vi "r3_Ladder bias ring encapsulation v1.vi"() -> ()   [LabVIEW 2016]
uses:
  WTF is this.ctl
  Classes/Controllers/I-O/Copy of NI-DAQ Folder/NI-DAQ.lvclass
  D:/INTT/V1/Classes/Controllers/I-O/Copy of I-O Folder/I-O.lvclass
  Classes/Controllers/Dispenser/Copy of Ultimus V2 Folder/Ultimus V2.lvclass
  <vilib>/Analysis/coordinate.llb/2D Cartesian Coordinate Rotation (Scalar).vi
  <vilib>/Utility/file.llb/Read Delimited Spreadsheet (DBL).vi
  <vilib>/Utility/file.llb/Write Delimited Spreadsheet (DBL).vi
  Classes/Controllers/Motion/Copy of Motion Folder/Motion.lvclass
  Classes/Controllers/Camera/Copy of Controller Folder/Controller.lvclass
  <vilib>/Analysis/NI_AALPro.lvlib
  Classes/Controllers/I-O/Copy of I-O Folder/I-O.lvclass
panel:
  in  "Needle gap for real":dbl=1.3
  out "corner index":i32
  out "Array":dbl[](array[numeric])
  out "x+y":dbl[](array[numeric])
  out "South":dbl[][][](array[numeric])
  out "North":dbl[][][](array[numeric])
  in  "deposit module":i32=2
  out "file indicator":dbl[][](array[numeric])
  out "?":dbl[](array[numeric]) format="%#_8g"
  in  "offset":dbl[](array[numeric])=[0.0, 0.0, 0.0, 0.0] format="%#_8g"
  out "HDI center positions":dbl[][](array[numeric]) format="%#_8g"
  out "HDI center positions":dbl[][](array[numeric])=[[459.92445114002015, 980.2358762511564, 78.77350133595746, 0.0015214873297426886]] format="%#_8g"
  out "CT sum up":dbl[](array[numeric])
  in  "txt switch":bool
  in  "MPT offset":dbl[][](array[numeric])=[[0.0, 0.0, 0.0, 0.0], [0.0, 0.0, 0.0, 0.0]] format="%#_8g"
  out "CT HPoS":dbl[][](array[numeric]) format="%#_8g"
  out "chip distance by OGP":dbl format="%#_8g"
  out "displacement":dbl[](array[numeric])
  out "gantry position test":dbl[](array[numeric])
  out "gantry target position":dbl[](array[numeric])
  out "chip distance by gantry":dbl format="%#_8g"
  out "after SL":dbl[](array[numeric]) format="%#_8g"
  out "after SR":dbl[](array[numeric]) format="%#_8g"
  out "after NL":dbl[](array[numeric]) format="%#_8g"
  out "S chip":dbl[](array[numeric]) format="%#_8g"
  out "N chip":dbl[](array[numeric]) format="%#_8g"
  in  "?":path=path "C:/Users/PAGANIS/Desktop/shih cheng wei/OGP/test1-2.txt"
  out "bless from OGP !!! Center of  stave":dbl[](array[numeric])
  out "bless from OGP !! measured stave size":dbl[](array[numeric])
  in  "Bless from OGP":bool
  out "FROM Detail !!! Center of module on stave":dbl[](array[numeric])
  out "FROM Detail !! measured stave size":dbl[](array[numeric])
  in  "Align Stave in detail":bool
  in  "check height?":bool
  in  "Uttimus presssure":i64=10
  out "Status":bool
  out "measured HDI top-left position":dbl[][](array[numeric])
  in  "HDI vacuum channel":i32=18
  in  "vacuum":bool=TRUE
  in  "HDI vacuum":bool
  out "measured stave size":dbl[](array[numeric])
  out "Stave mark":dbl[][](array[numeric])
  out "Center of module on stave":dbl[](array[numeric])
  out "Measured HDI size":dbl[][](array[numeric])
  out "MPT positions on stave":T1[][](array[typedef])
  in  "Default Stave dimension":dbl[](array[numeric])=[34.0, 472.0, -0.335295, -0.000320234]
  in  "Default Stave upper left mark":dbl[](array[numeric])=[584.376, 675.576, 70.9882, 0.000840064]
  out "Needle parking position":dbl[](array[numeric])
  in  "Uppler / Lower Stave":bool=TRUE
  out "Gantry current position":dbl[](array[numeric])
  in  "READ Position":bool
  in  "Needle Height Compenstation\n(glue gap)":dbl=0.33
  in  "Needle Alignment":bool
  in  "Parking position":dbl[](array[numeric])=[625.0, 625.0, 0.0, 0.01]
  in  "GOTO":bool
  in  "Default Pickup Tool Position":dbl[][](array[numeric])=[[152.226, 682.729, 36.8129, -0.0151898], [700.0, 800.0, 20.0, 0.01]]
  in  "deposit glue module":i32=1
  in  "Default HDI alignment \nmark position":dbl[](array[numeric])=[589.244, 676.291, 66.3411, 0.000190613]
  in  "Default HDI size":dbl[](array[numeric])=[24.2437, 231.446, -0.099339, 0.000191129]
  out "# of tasks excuted":i32
  out "PickupTool \nCenterPosition":dbl[](array[numeric]) format="%#_8g"
  in  "Inititalize":bool
  in  "Pick and place":bool
  in  "Deposit Glue":bool
  in  "Measure Pickup Tools":bool
  in  "Align Stave":bool
  out "default module position on stave":dbl[][](array[numeric])
  in  "Stop":bool
  in  "Measure HDI":bool
  # "Ladder Assembly"
  # "To switch the north/south\ntxt file \nswitch \noffset\nmodule pick up tool\nmodule direction"
  # "Upper\nmodule"
  # "Lower\nmodule"
  # "Sensor 0.32 -> 200 micron glue thickness\nChips 0.37-> 140 micron glue thickness"
  # "ACTIONS"
  # "theta had *-1"
  # "Pick up tool and needle"
  # "Module infomation"
  # "Pick and Place"
  # "CT"
  # "+"
  # "+"
  # "="
  # "Bias ring encapsulation"
  # "before \"HDI cornrer\" click \"Initialize\""
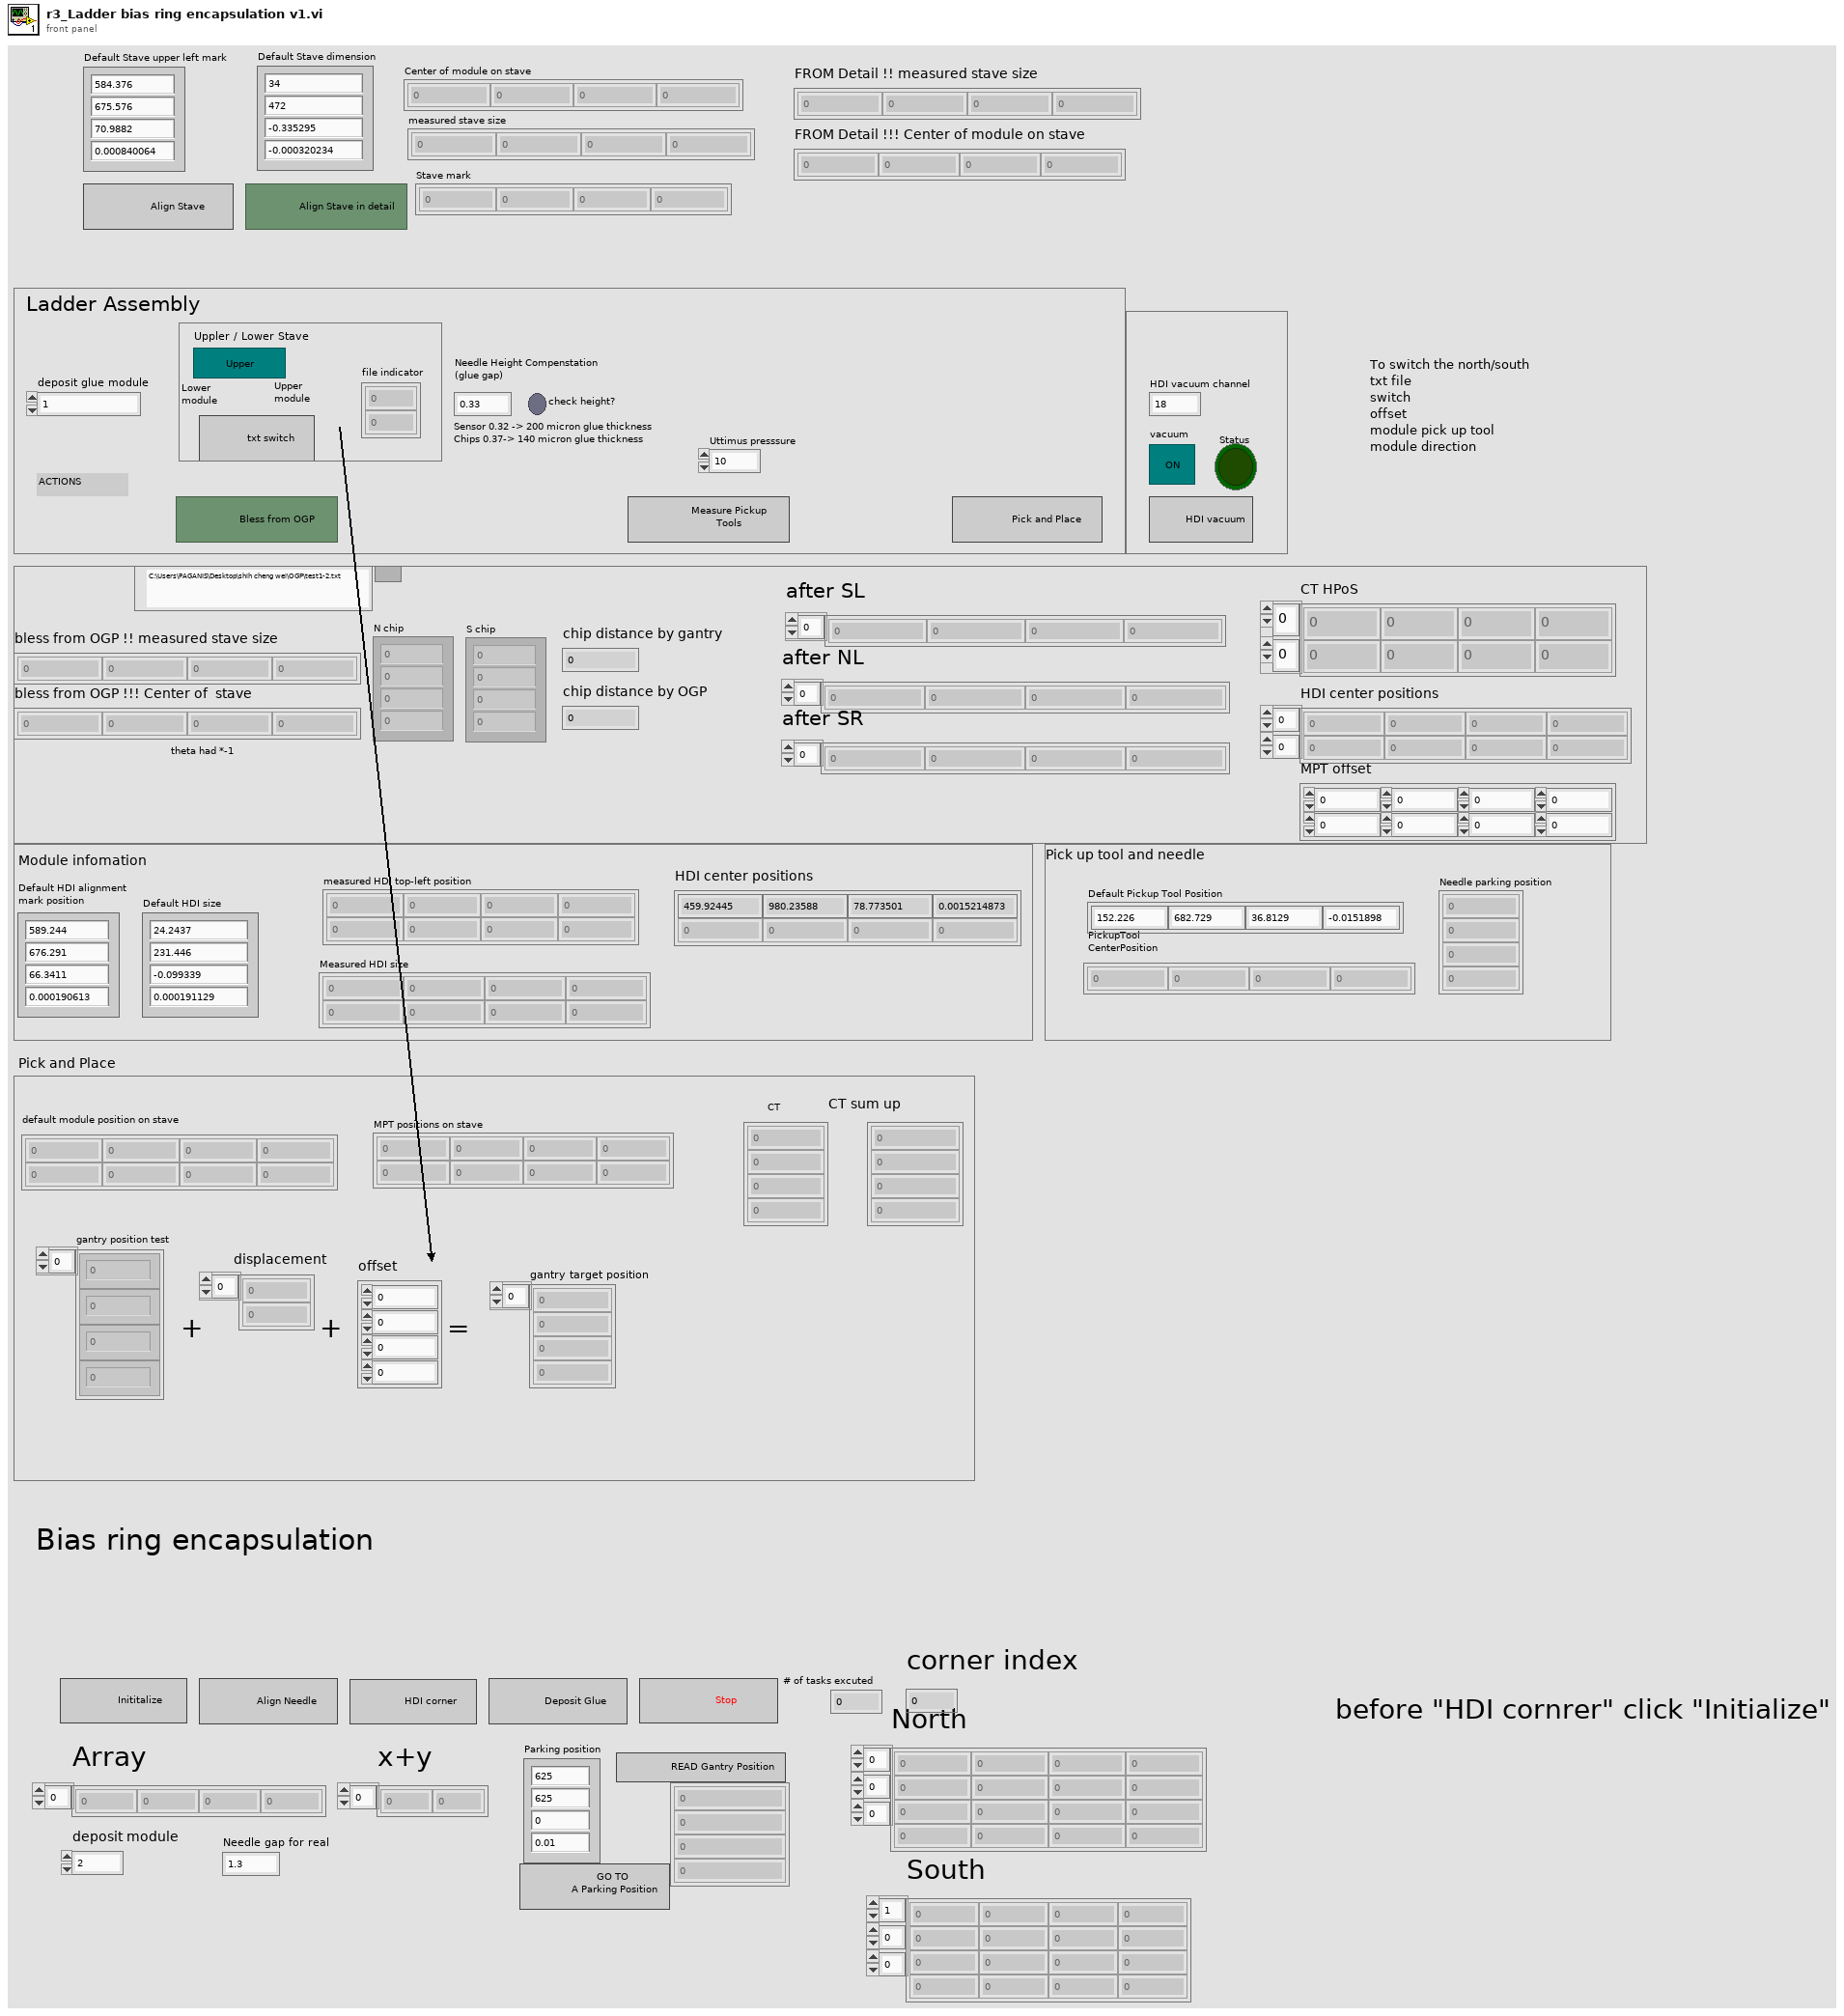
[diagram p1: front panel]
types:
  T1 = typedef "WTF is this.ctl" = dbl
  T2 = typedef "Controller.lvclass/Controllers.ctl" = cluster{"Copy of Motion.lvclass":refnum<class "Motion.lvclass">, "Copy of I-O.lvclass":refnum<class "I-O.lvclass">, "Copy of Dispenser.lvclass":refnum<class "Dispenser.lvclass">}
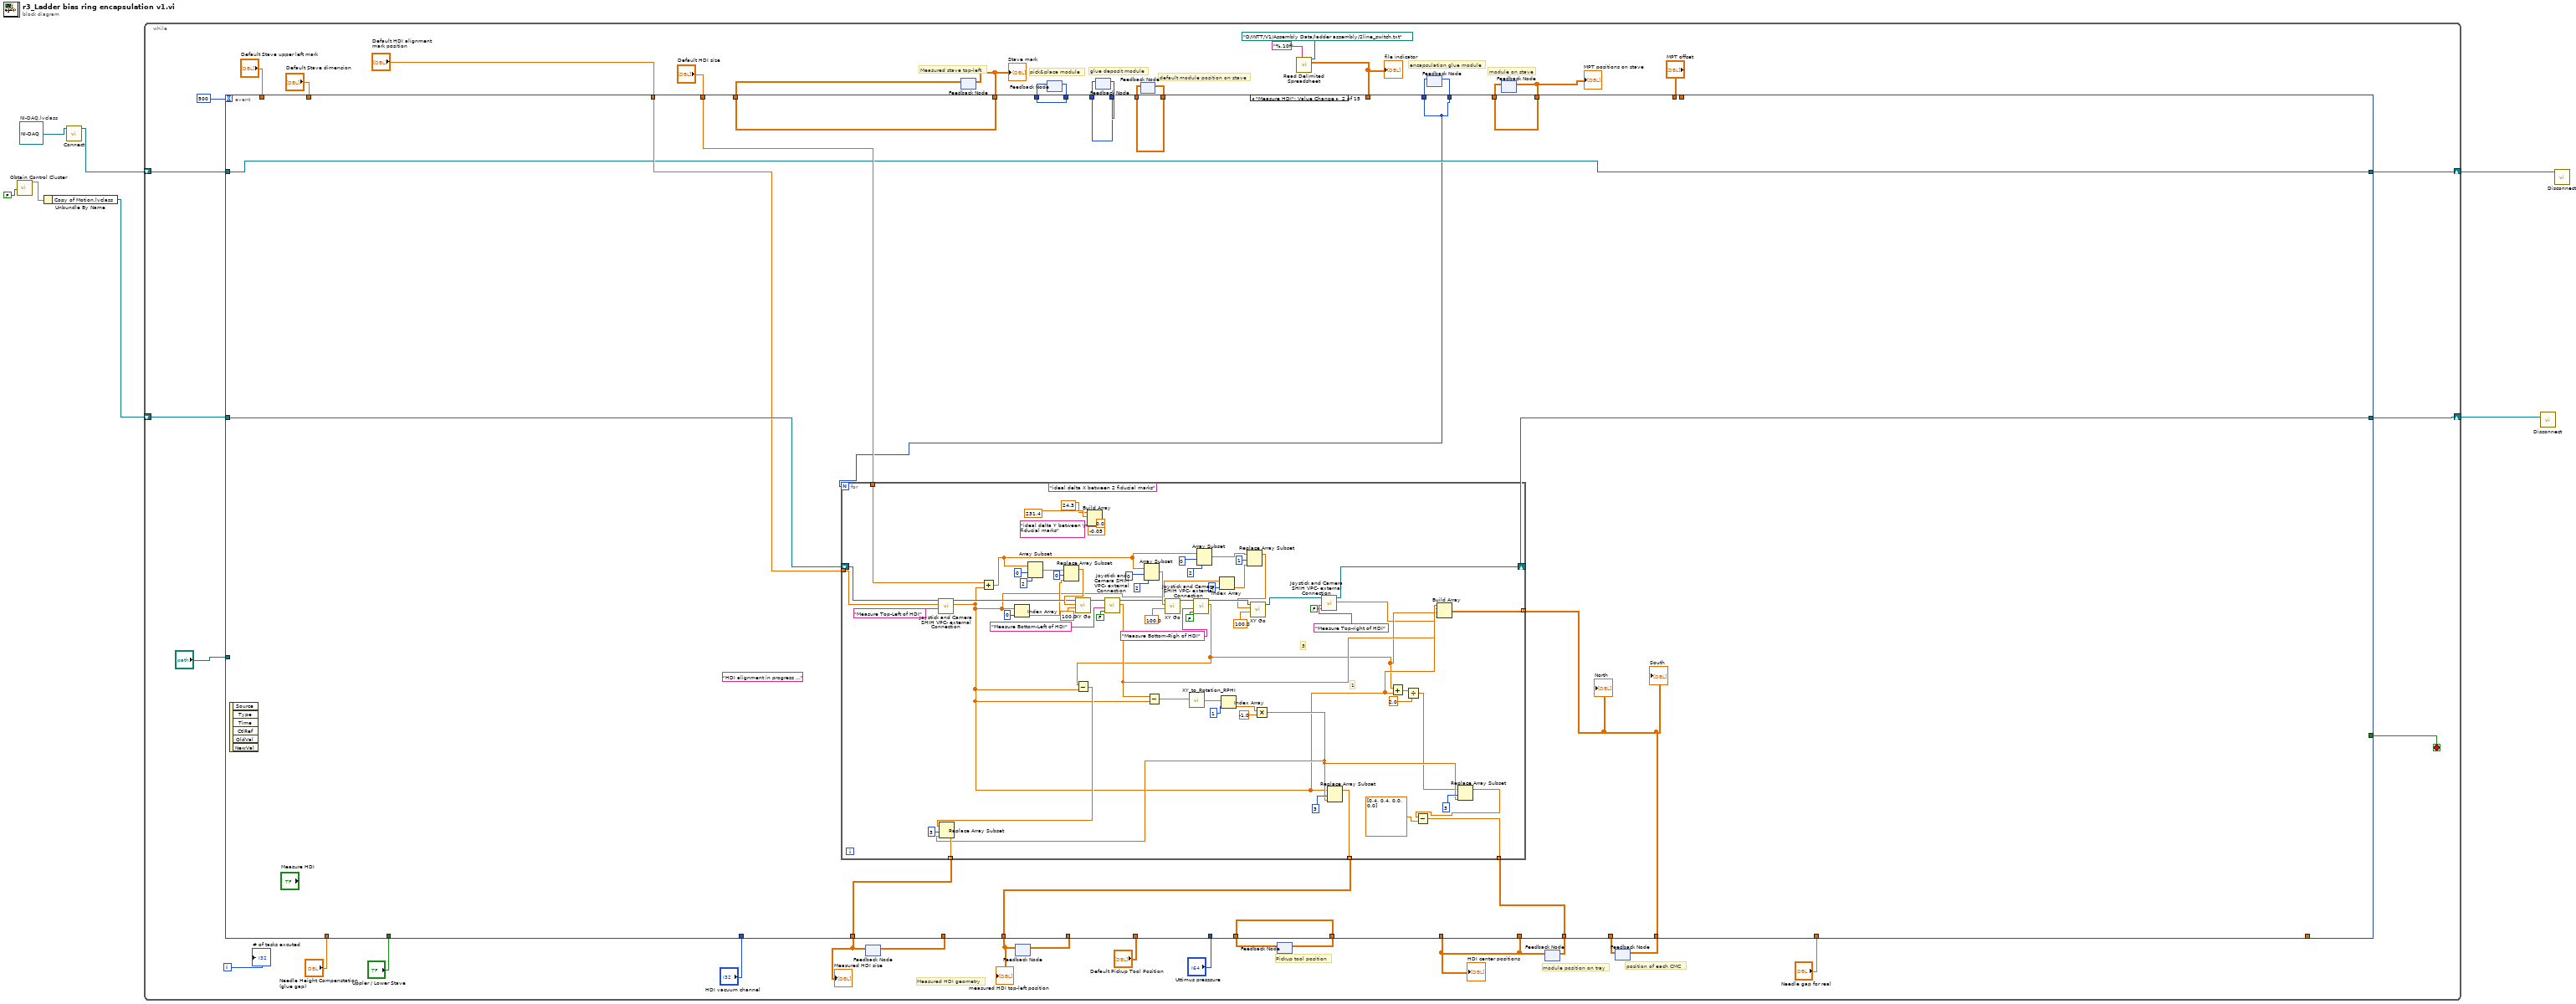
[diagram p0: block diagram]
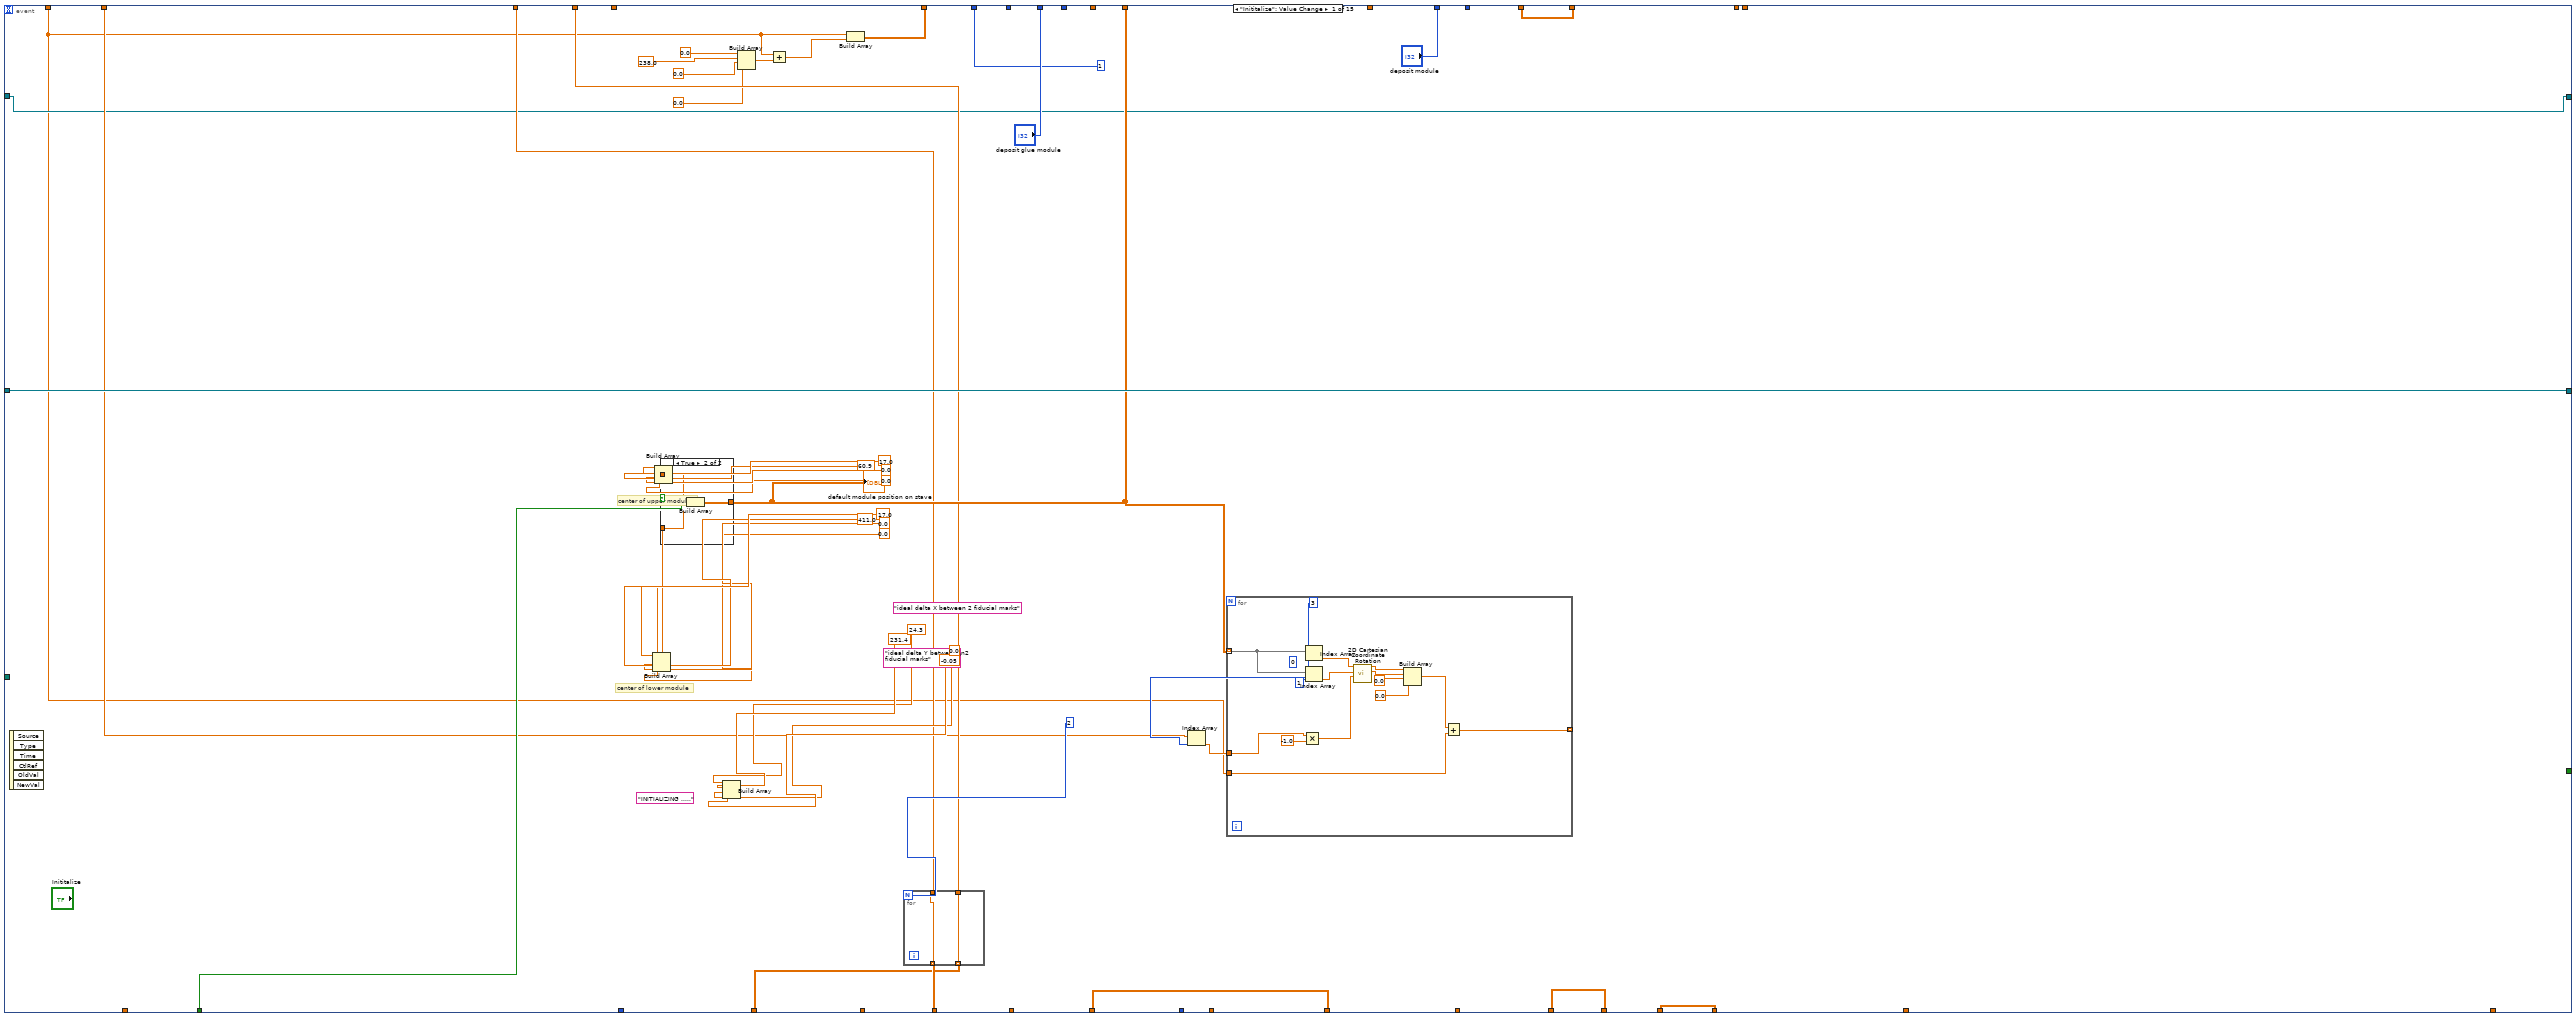
[diagram p2: hidden frame]
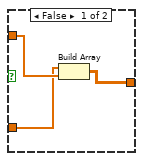
[diagram p3: hidden frame]
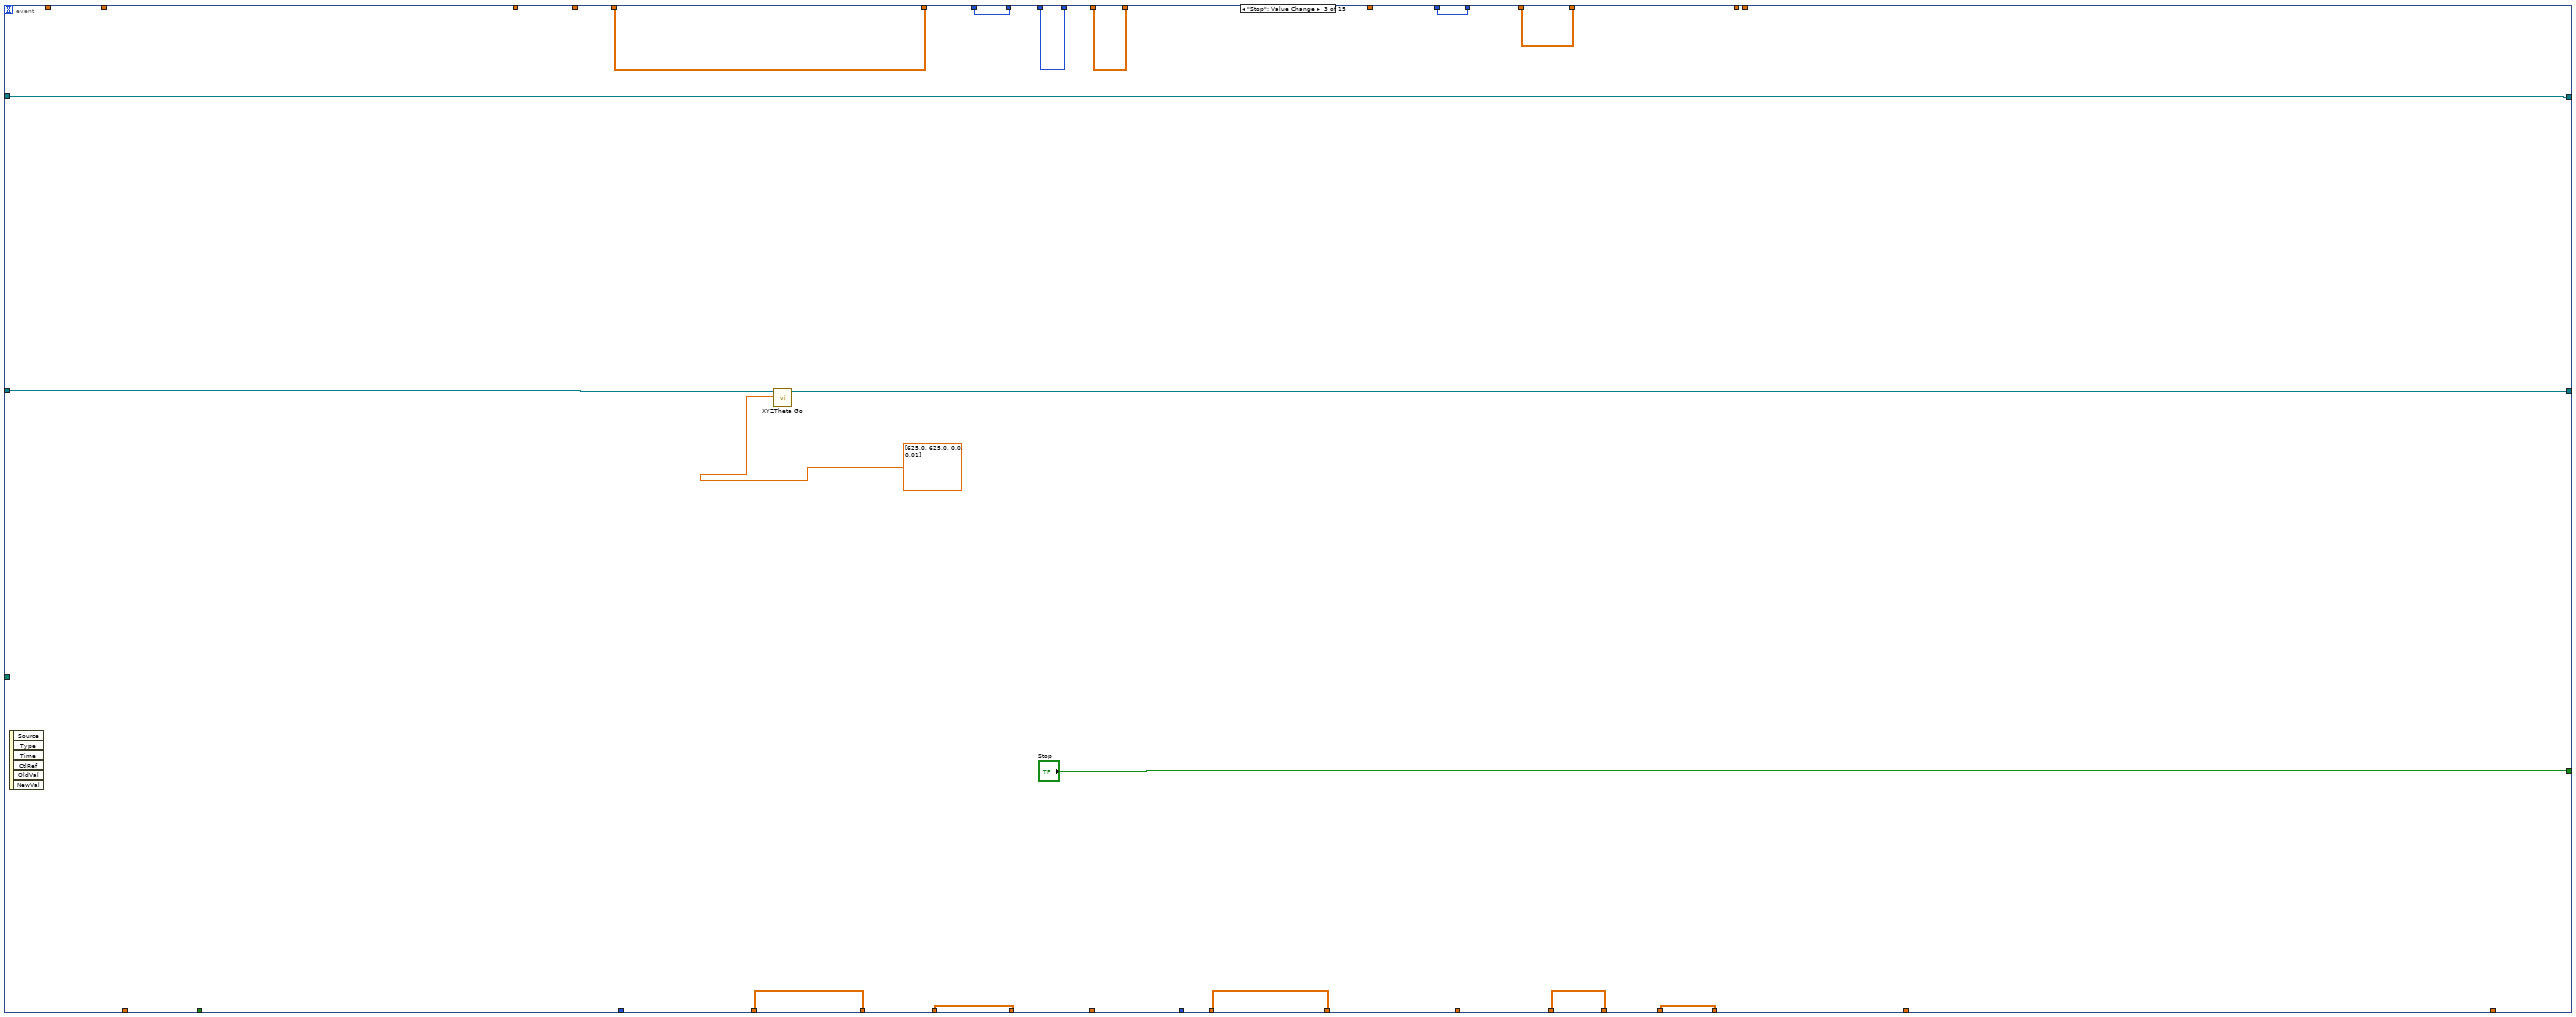
[diagram p4: hidden frame]
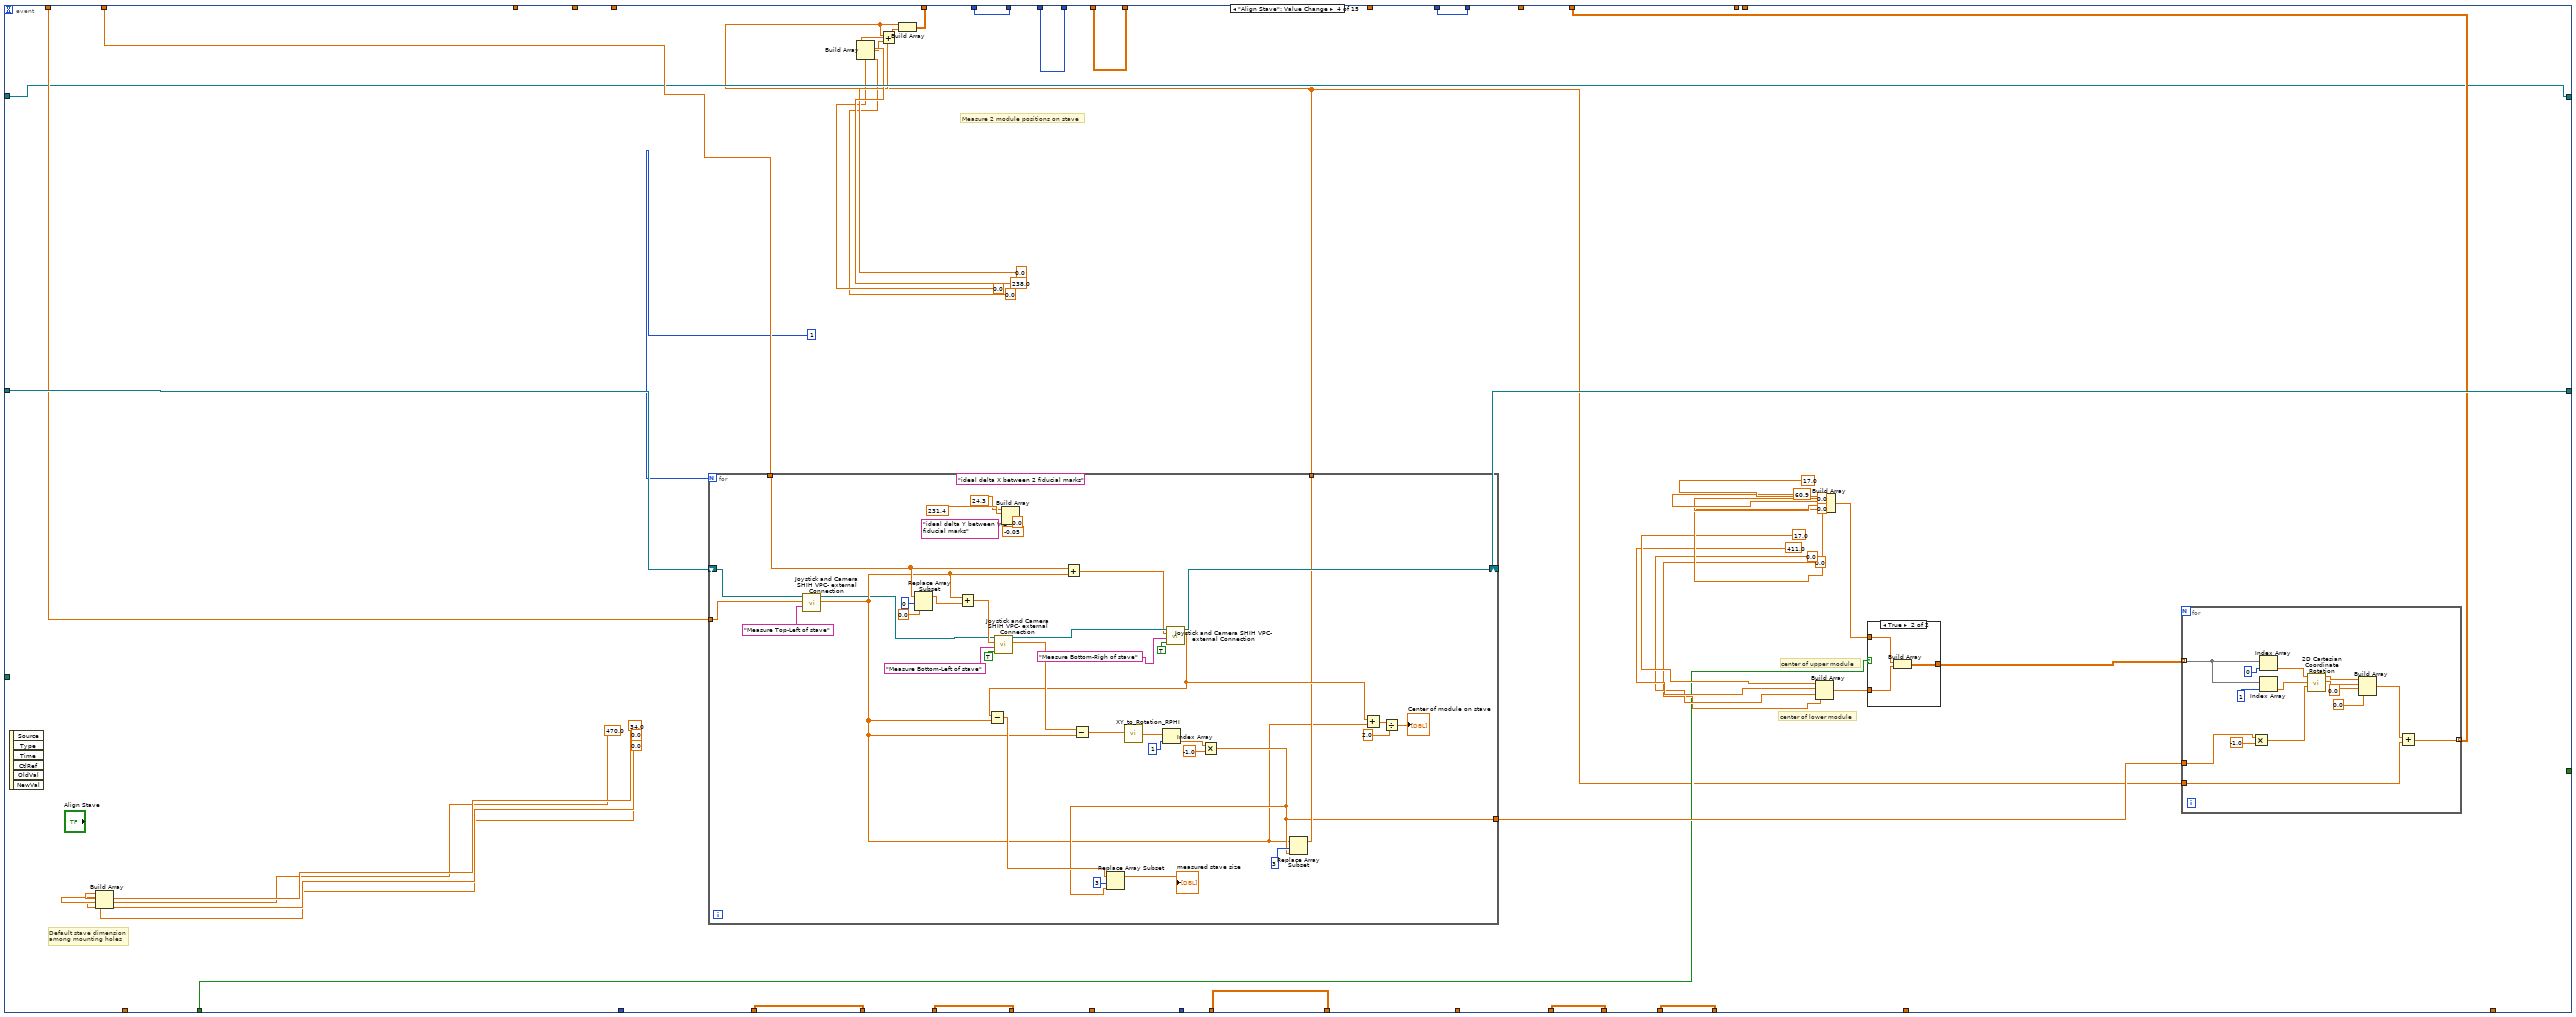
[diagram p5: hidden frame]
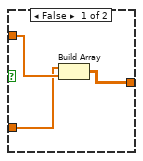
[diagram p6: hidden frame]
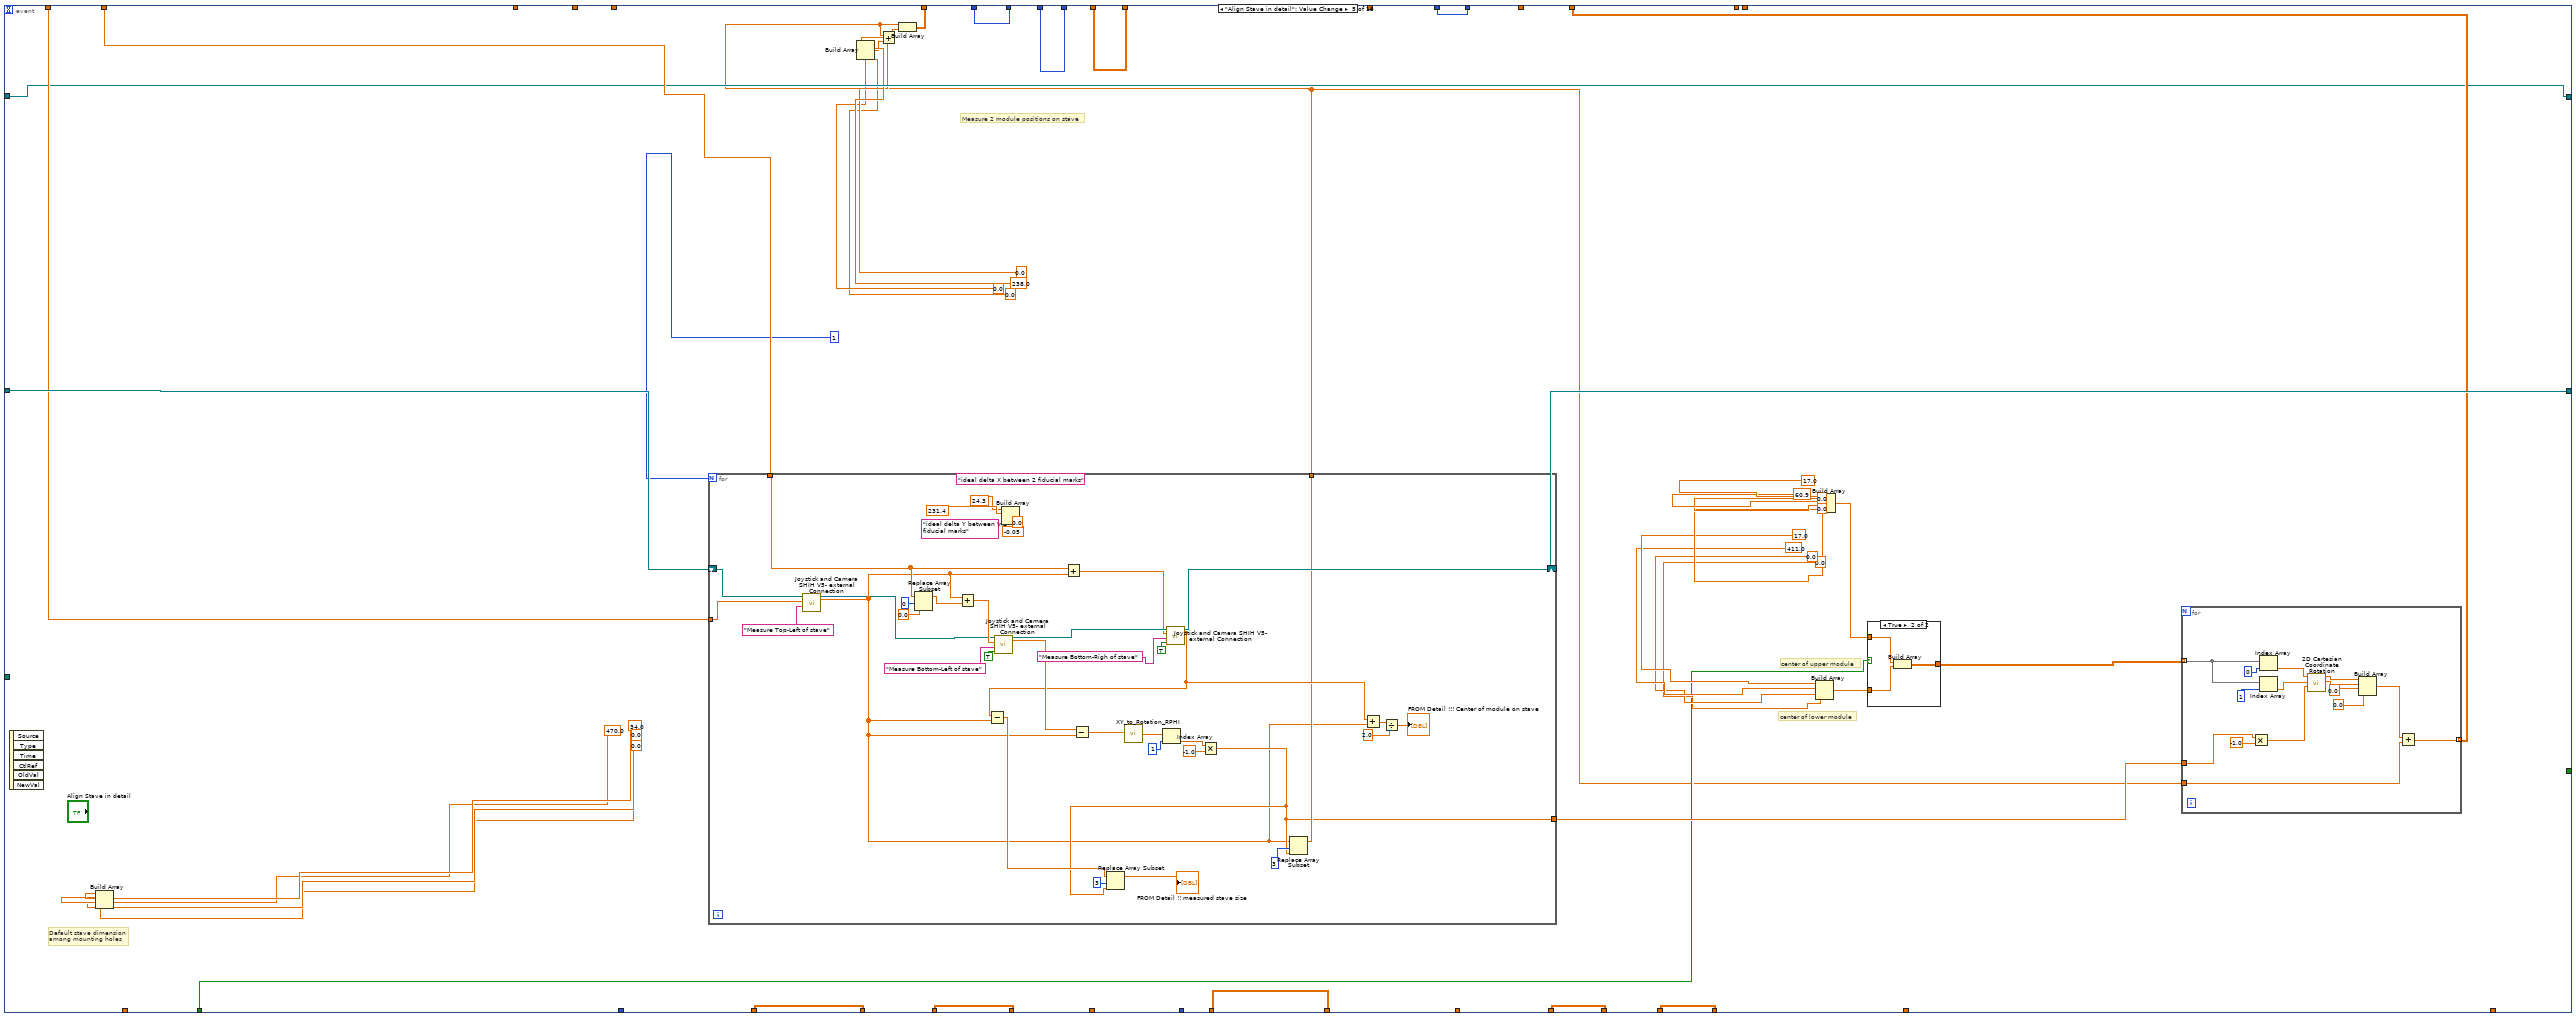
[diagram p7: hidden frame]
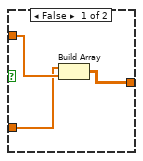
[diagram p8: hidden frame]
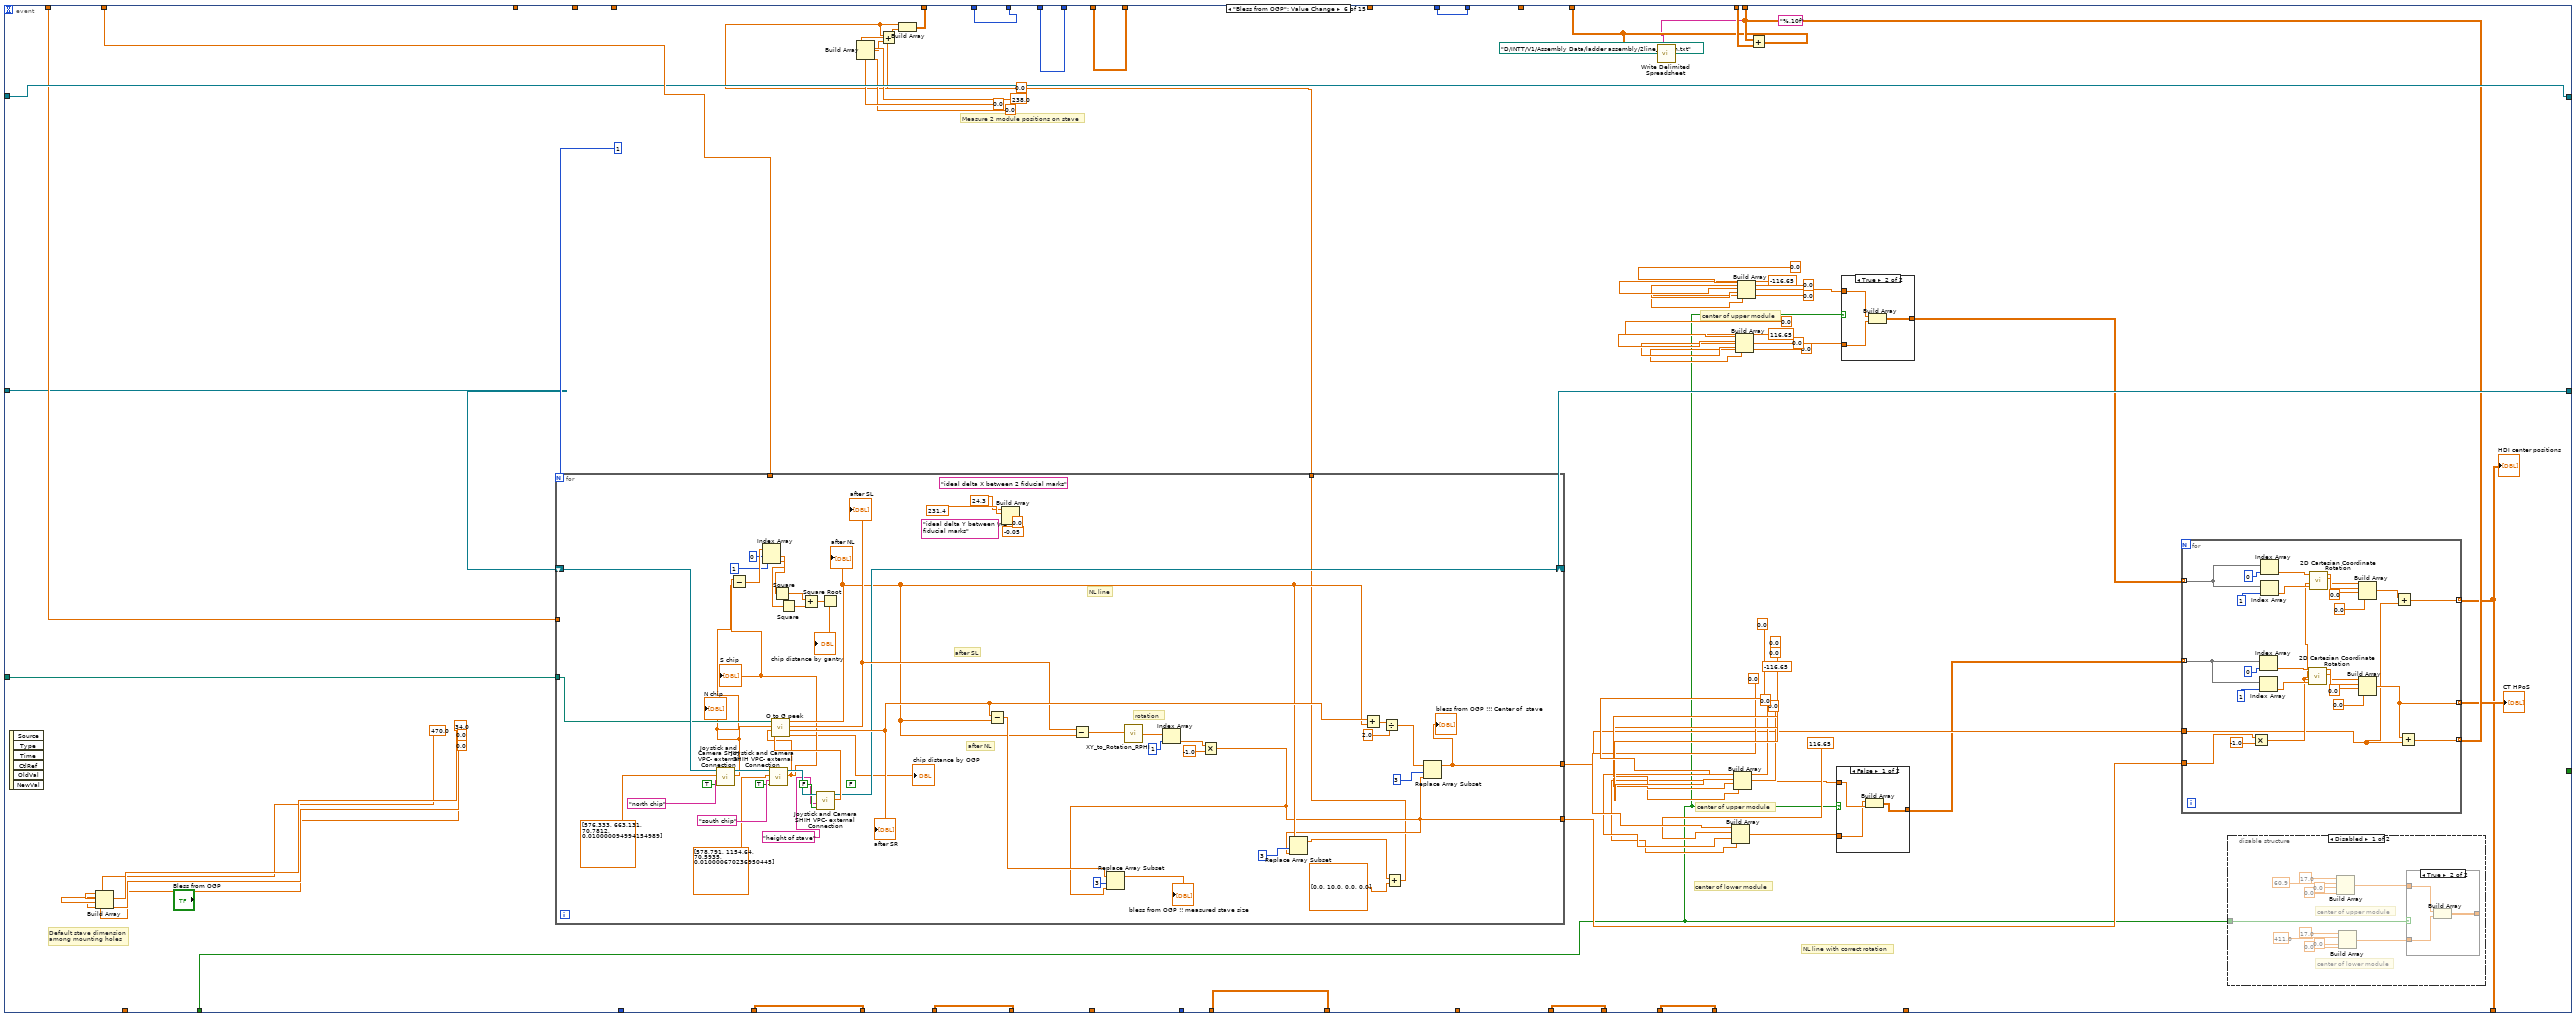
[diagram p9: hidden frame]
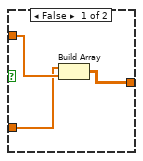
[diagram p10: hidden frame]
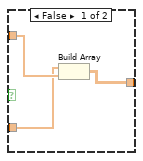
[diagram p11: hidden frame]
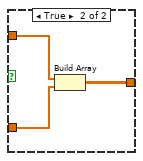
[diagram p13: hidden frame]
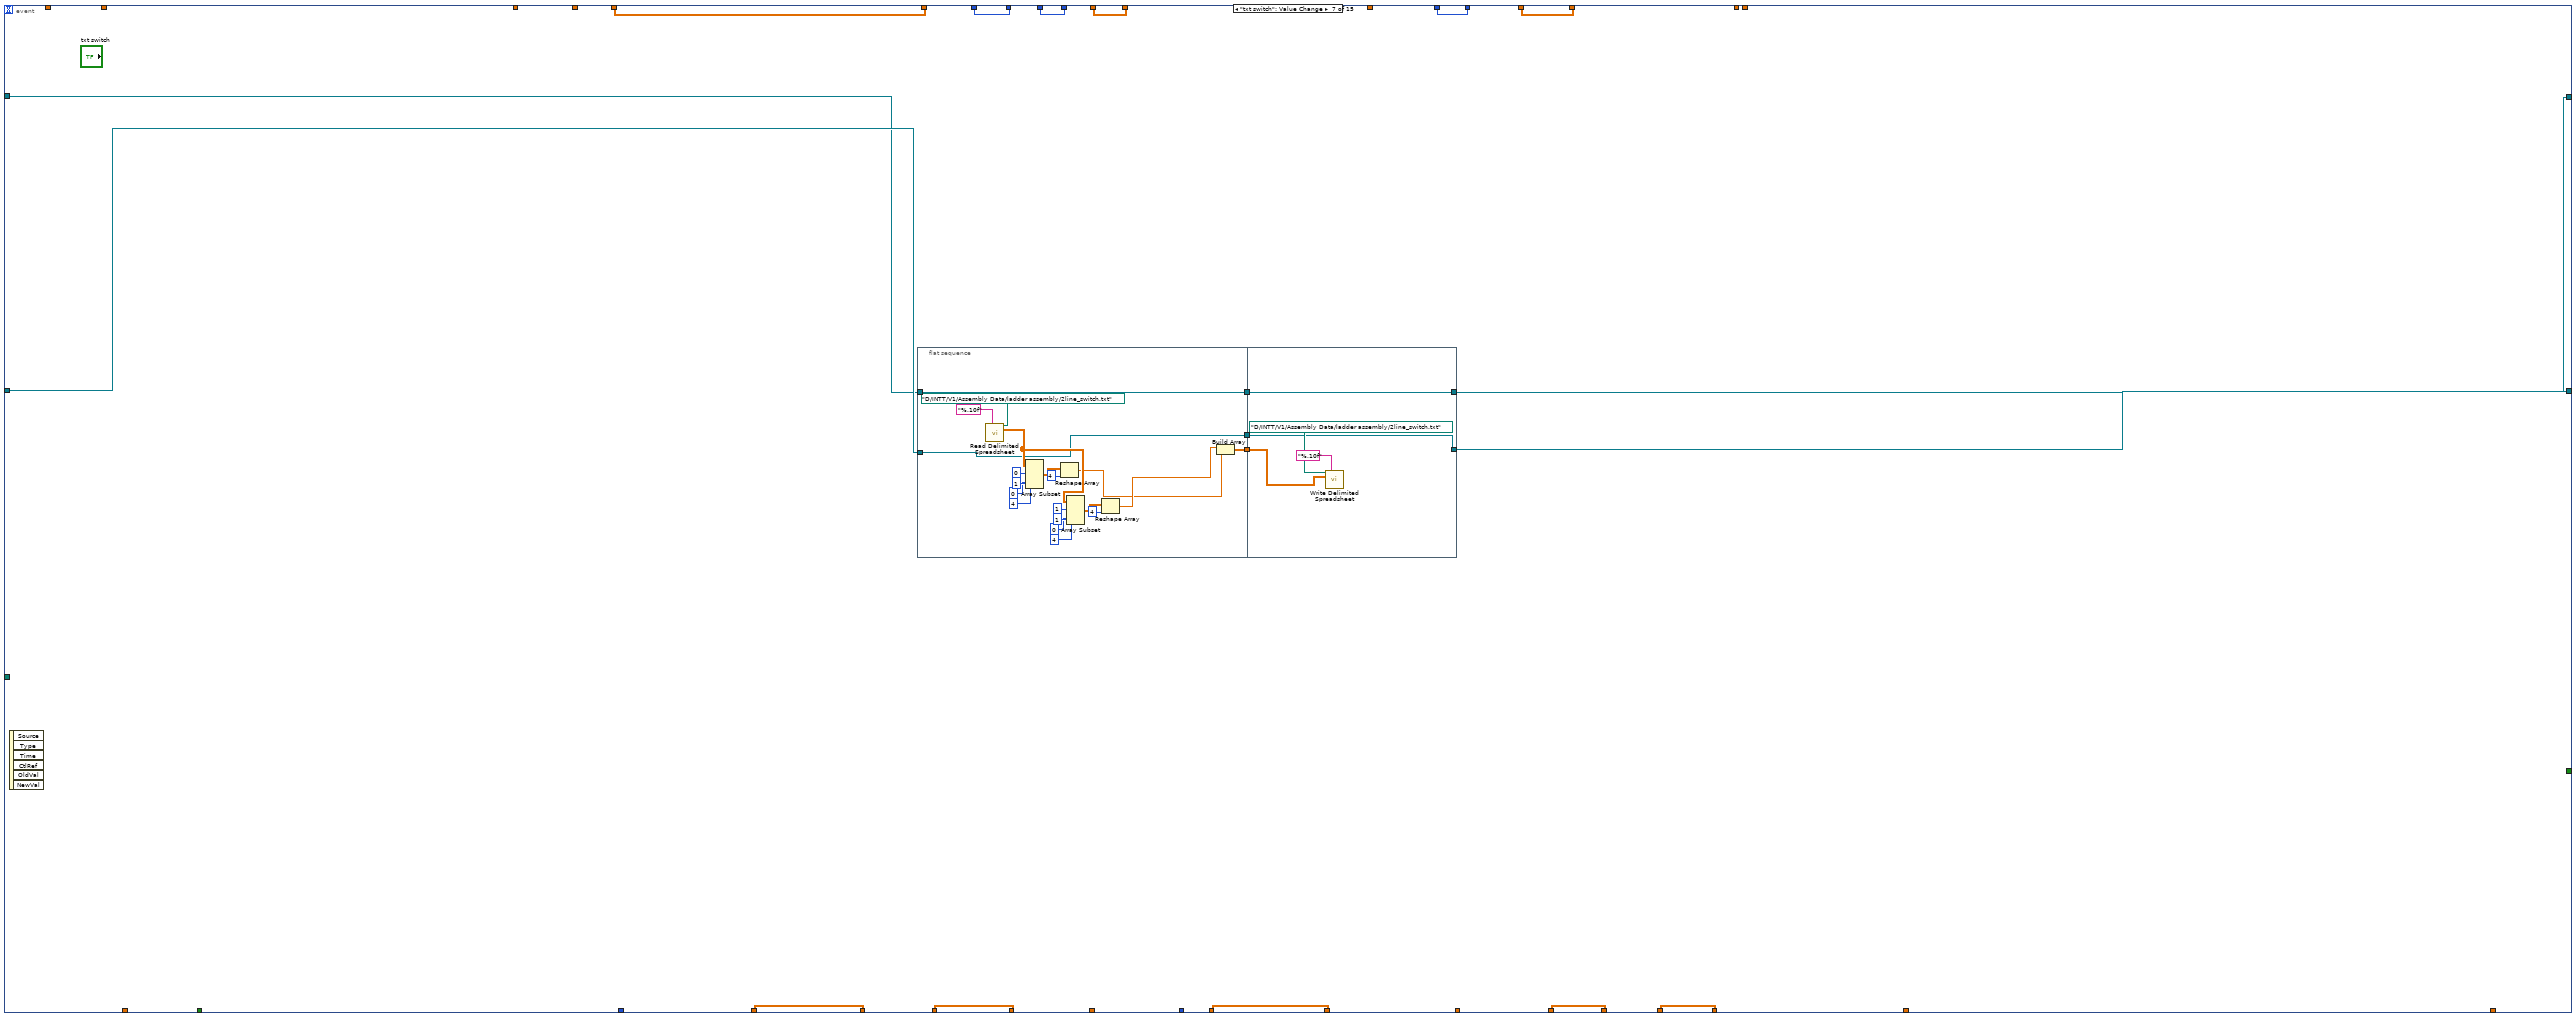
[diagram p14: hidden frame]
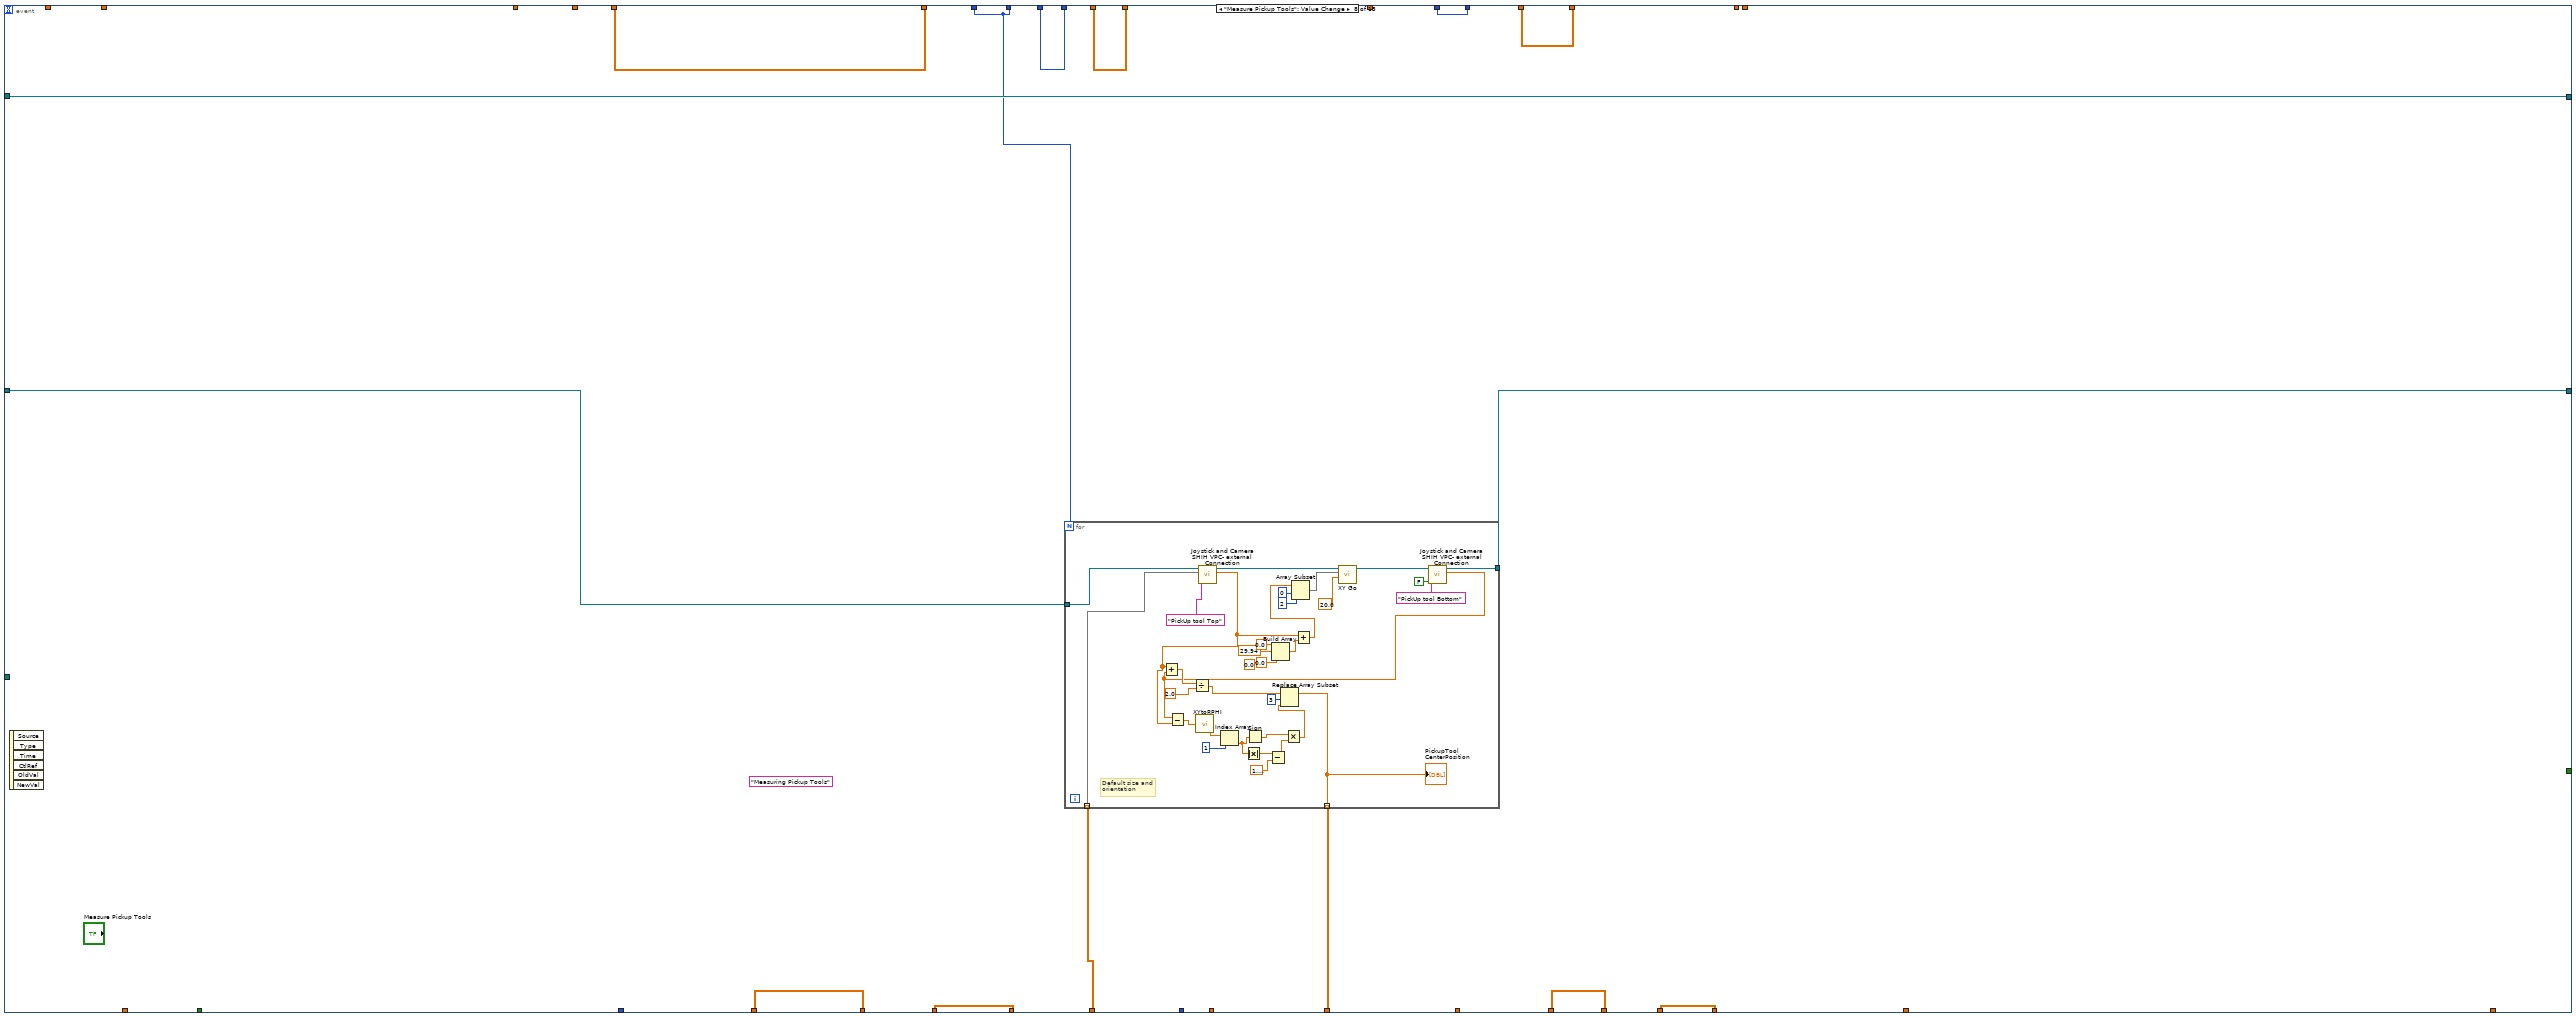
[diagram p15: hidden frame]
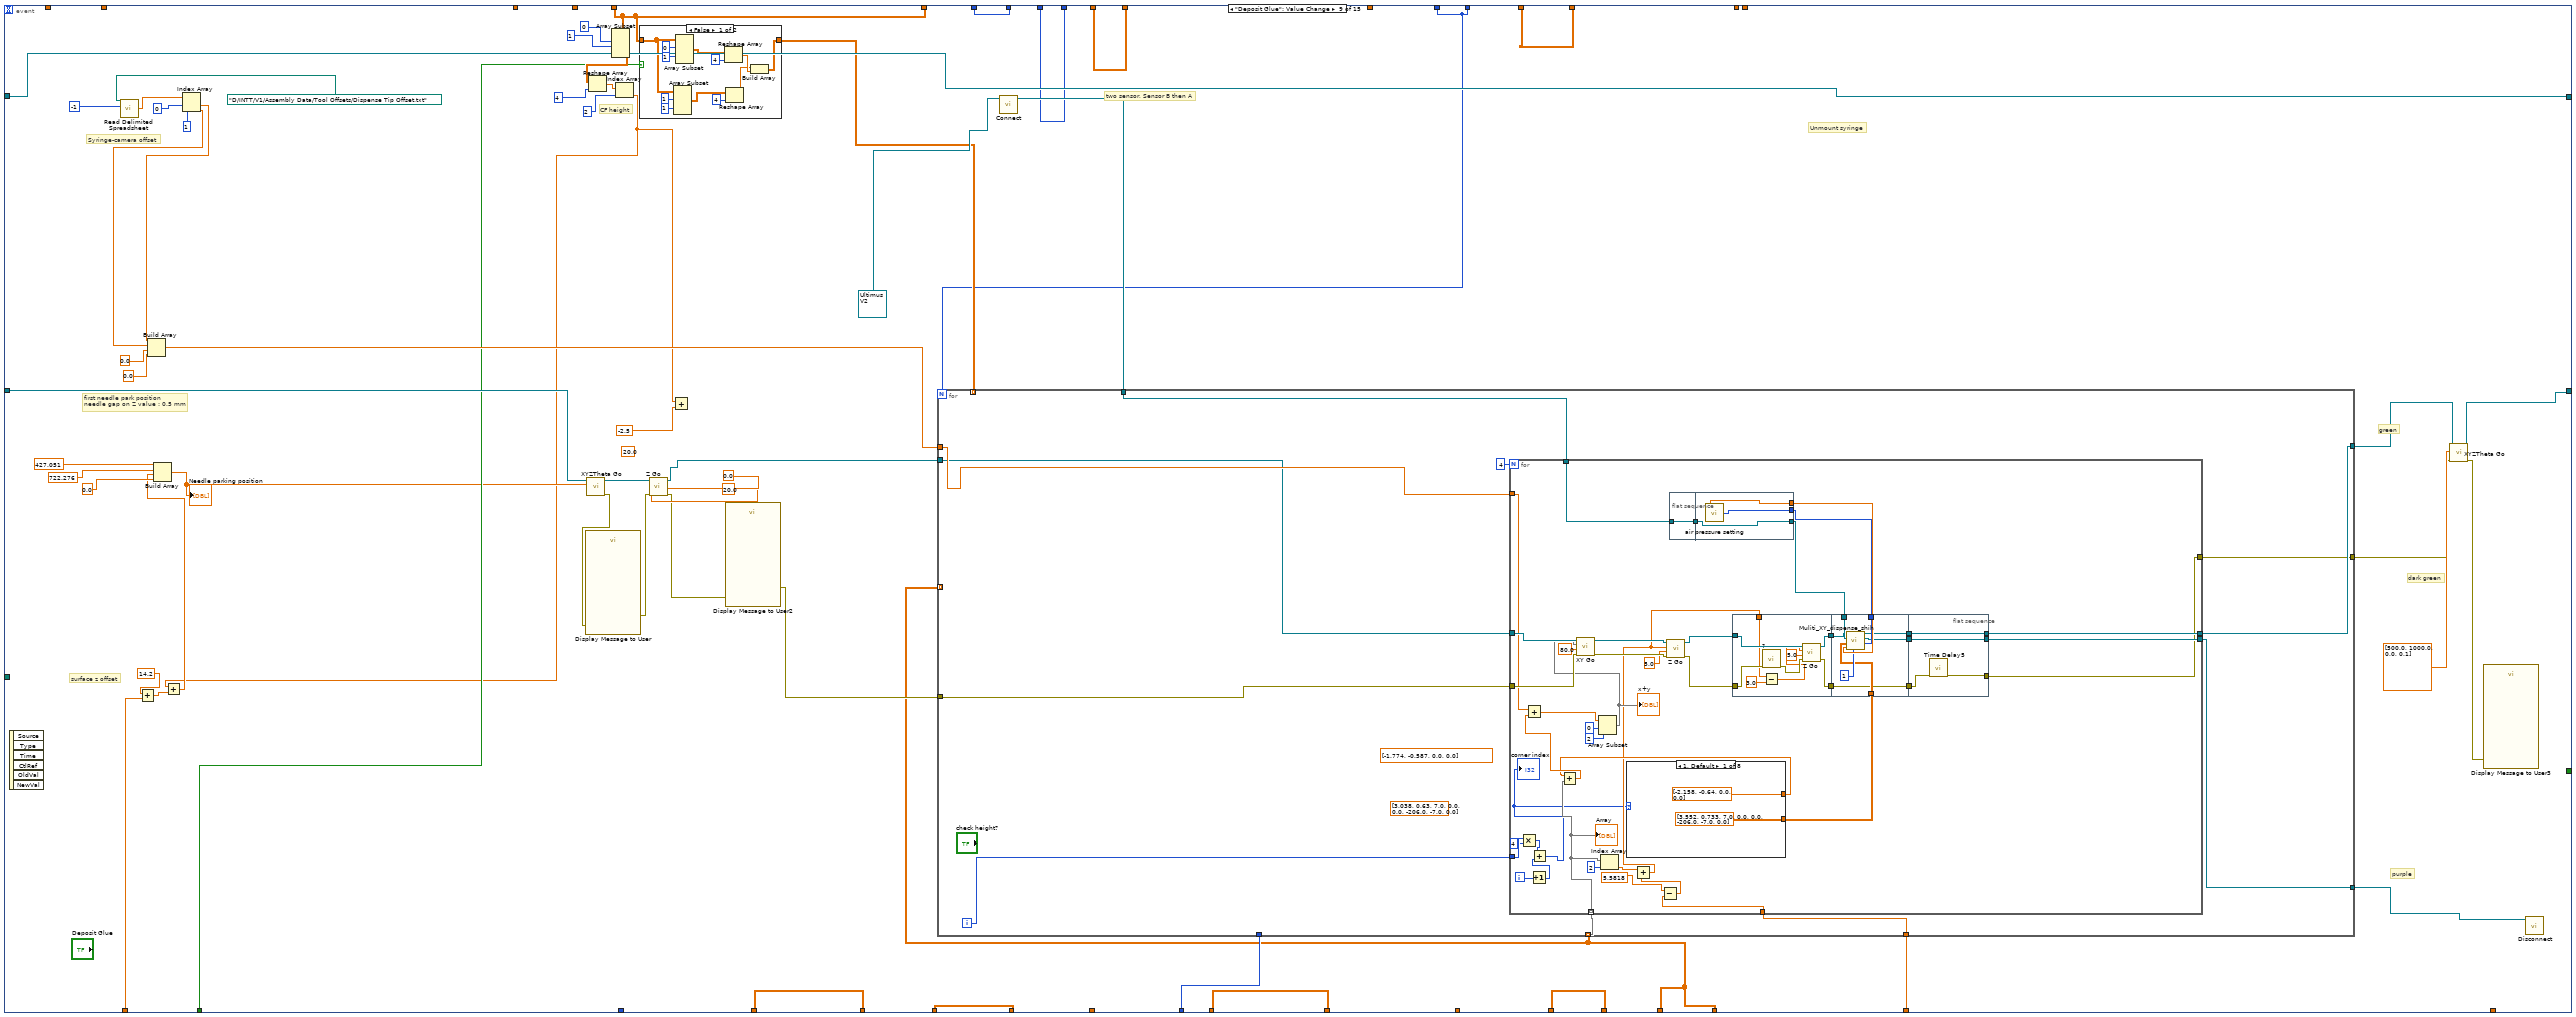
[diagram p16: hidden frame]
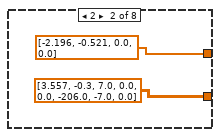
[diagram p18: hidden frame]
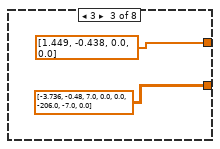
[diagram p19: hidden frame]
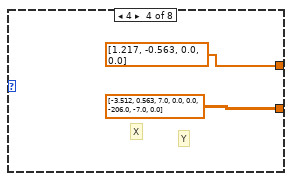
[diagram p20: hidden frame]
diagram:
  w3 = refnum<class "NI-DAQ.lvclass"> refnum  # NI-DAQ.lvclass
  n1 = call "Obtain Control Cluster.vi"("I/O"=FALSE) -> ("Control Out"=w7:T2)  [unwired: 10 in]
  n2 = Unbundle By Name(w7) -> ("Copy of Motion.lvclass"=w5:refnum<class "Motion.lvclass">)
  n3 = call-dynamic "Connect.vi"("NI-DAQ in"=w3) -> ("NI-DAQ out"=w2:refnum<class "NI-DAQ.lvclass">)  [unwired: 9 in, 1 out]
  n4 = while {
    shift-right: [w44] -> w4
    shift-left: w5 -> [w51]
    shift-right: [w24] -> w1
    shift-left: w2 -> [w28]
    i -> [w43]
    stop <- w50 stop-if-true
    # "position of each CMC"
    # "encapsulation glue module"
    # "pick&place module"
    # "default module position on stave"
    # "Pickup tool position"
    # "glue deposit module"
    # "Measured HDI geometry"
    # "module position on tray"
    # "Measured stave top-left"
    # "module on stave"
    n5 = feedback #1() -> (w48:dbl[][])  [unwired: 1 in]
    n6 = feedback #2() -> (w49:dbl[][])  [unwired: 1 in]
    n7 = feedback #3() -> (w25:dbl[][])  [unwired: 1 in]
    n8 = feedback #4() -> (w14:i32)  [unwired: 1 in]
    n9 = feedback #5() -> (w42:i32)  [unwired: 1 in]
    n10 = feedback #6() -> (w37:dbl[][])  [unwired: 1 in]
    n11 = feedback #7() -> (w45:dbl[][])  [unwired: 1 in]
    n12 = call-poly <vilib>:"Read Delimited Spreadsheet.vi"("file path (dialog if empty)"=path "D:/INTT/V1/Assembly Data/ladder assembly/2line_switch.txt" ("file path (dialog if empty) 3"), "format (%.3f)"="%.10f") -> ("all rows"=w16:dbl[][])  [unwired: 8 in, 5 out]
    "file indicator" <- w16
    n13 = feedback #8() -> (w11:i32)  [unwired: 1 in]
    n14 = feedback #9() -> (w32:dbl[][])  [unwired: 1 in]
    n15 = feedback #10() -> (w13:dbl[][])  [unwired: 1 in]
    "HDI center positions" <- w13
    n16 = feedback #11() -> (w9:dbl[][][])  [unwired: 1 in]
    n17 = event shown="[1] \"Measure HDI\": Value Change" {
      selector: _ -> [_ _ _ _ _ _ _ _ _ _ _ _ _ _ _]
      dyn-events: _ -> [_ _ _ _ _ _ _ _ _ _ _ _ _ _ _]
      timeout: 500 -> [_ _ _ _ _ _ _ _ _ _ _ _ _ _ _]
      tunnel: w51 -> [w88 w130 w211 w244 w343 w444 w583 w633 w709 w873 w940 w1105 w1126 w1131 w1155]
      tunnel: [_ _ "Stop" _ _ _ _ _ _ _ _ _ _ _ _] -> w50
      tunnel: [w56 w124 w206 w215 w314 w447 w588 w628 w676 w839 w921 w1111 w1122 w1139 w1154] -> w29
      tunnel: w49 -> [_ w124 w206 _ _ _ w588 w628 w676 w839 w921 w1111 w1122 w1139 w1154]
      tunnel: [w66 w122 w205 w240 w339 w459 w592 w627 w698 w876 w923 w1108 w1121 w1133 w1152] -> w30
      tunnel: w48 -> [_ _ w205 w240 w339 w459 w592 w627 w698 w876 w923 w1108 w1121 w1133 w1152]
      tunnel: w42 -> [_ w117 w208 w245 w344 w462 w587 w624 w672 w878 w917 w1110 w1123 w1137 w1146]
      tunnel: [w71 w121 w203 w247 w346 w464 w589 w626 w700 w874 w908 w1106 w1119 w1135 w1149] -> w47
      tunnel: w13 -> [w71 _ w203 w247 w346 w464 w589 w626 w700 w874 w908 w1106 w1119 w1135 w1149]
      tunnel: [w86 w125 w204 w252 w351 w469 w590 w632 w699 w875 w929 w1107 w1120 w1134 w1150] -> w46
      tunnel: w45 -> [_ w125 w204 w252 w351 w469 w590 _ w699 w875 w929 w1107 w1120 w1134 w1150]
      tunnel: [w88 w129 w209 w241 w340 w460 w581 w631 w701 w865 w930 w1103 w1125 w1131 w1155] -> w44
      tunnel: ["deposit glue module" w117 w208 w245 w344 w462 w587 w624 w672 w878 w917 w1110 w1123 w1137 w1146] -> w41
      tunnel: "Default HDI alignment \nmark position" -> [w69 w128 _ _ _ _ _ _ _ _ _ _ _ _ _]
      tunnel: "Default HDI size" -> [w68 w127 _ _ _ _ _ _ _ _ _ _ _ _ _]
      tunnel: [w75 w126 w207 w246 w345 w463 w586 w629 w697 w877 w928 w1109 w1124 w1138 w1153] -> w38
      tunnel: w37 -> [_ w126 w207 w246 w345 w463 w586 w629 w697 w877 w928 w1109 w1124 w1138 w1153]
      tunnel: "Default Pickup Tool Position" -> [w86 _ _ _ _ _ _ w630 _ _ _ _ _ _ _]
      tunnel: "Uppler / Lower Stave" -> [w72 _ _ w225 w324 w414 _ _ w684 _ w897 _ _ _ _]
      tunnel: "Default Stave upper left mark" -> [w57 _ _ w243 w342 w446 _ _ _ _ _ _ _ _ _]
      tunnel: "Default Stave dimension" -> [w65 _ _ w242 w341 w461 _ _ _ _ _ _ _ _ _]
      tunnel: [w54 w123 w201 w224 w323 w428 w585 w625 w696 w856 w919 w1101 w1116 w1136 w1148] -> w31
      tunnel: w32 -> [w54 w123 w201 _ _ _ w585 w625 w696 w856 w919 w1101 w1116 w1136 w1148]
      tunnel: w28 -> [w64 w119 w199 w223 w322 w455 w580 w622 w691 w854 w926 w1100 w1115 w1143 w1158]
      tunnel: [w64 w119 w199 w223 w322 w455 w578 w622 w691 w854 w925 w1100 w1115 w1130 w1156] -> w24
      tunnel: "HDI vacuum channel" -> [_ _ _ _ _ _ _ _ _ _ w924 _ _ w1140 w1157]
      tunnel: [w67 w120 w200 w239 w338 w458 w591 w623 w692 w855 w922 w1102 w1117 w1132 w1151] -> w26
      tunnel: w25 -> [_ _ w200 w239 w338 w458 w591 w623 w692 w855 w922 w1102 w1117 w1132 w1151]
      tunnel: "Needle Height Compenstation\n(glue gap)" -> [_ _ _ _ _ _ _ _ w686 w847 _ _ _ _ _]
      tunnel: "Uttimus presssure" -> [_ _ _ _ _ _ _ _ w685 _ _ _ _ _ _]
      tunnel: "?" -> [_ _ _ _ _ w445 _ _ _ _ _ _ _ _ _]
      tunnel: [_ _ _ _ _ w443 _ _ _ _ _ _ _ _ _] -> _
      tunnel: "MPT offset" -> [_ _ _ _ _ w429 _ _ _ _ _ _ _ _ _]
      tunnel: w16 -> [_ _ _ _ _ _ _ _ _ _ w920 _ _ _ _]
      tunnel: [1 ("pick &place module") w118 w198 w214 w313 w425 w584 w621 w675 w837 w918 w1099 w1114 w1129 w1147] -> w15
      tunnel: w14 -> [_ w118 w198 w214 w313 w425 w584 w621 w675 w837 w918 w1099 w1114 w1129 w1147]
      tunnel: w13 -> [_ _ _ _ _ _ _ _ _ _ w898 _ _ _ _]
      tunnel: [_ _ _ _ _ w412 _ _ _ _ _ _ _ _ _] -> _
      tunnel: ["deposit module" w116 w197 w213 w312 w411 w577 w620 w673 w836 w894 w1098 w1113 w1128 w1145] -> w12
      tunnel: w11 -> [_ w116 w197 w213 w312 w411 w577 w620 w673 w836 w894 w1098 w1113 w1128 w1145]
      tunnel: [w52 w115 w196 w212 w311 w410 w576 w619 w668 w835 w893 w1097 w1112 w1127 w1144] -> w10
      tunnel: w9 -> [w52 _ w196 w212 w311 w410 w576 w619 w668 w835 w893 w1097 w1112 w1127 w1144]
      tunnel: "Needle gap for real" -> [_ _ _ _ _ _ _ _ w669 _ _ _ _ _ _]
      event "Inititalize": Value Change {
        (unwired) "INITIALIZING ....." ("String")
        (unwired) "ideal delta Y between \n2 fiducial marks"
        (unwired) "ideal delta X between 2 fiducial marks"
        # "center of lower module"
        # "center of upper module"
        n18 = event-data() -> ()  [unwired: 1 in, 6 out]
        n19 = Build Array(17.0 ("element"), 411.0 ("element"), 0.0 ("element"), 0.0 ("element")) -> (w76:dbl[])
        n20 = Build Array(17.0 ("element"), 60.9 ("element"), 0.0 ("element"), 0.0 ("element")) -> (w77:dbl[])
        n21 = case shown="True" w72 {
          tunnel: w77 -> [w97 w100]
          tunnel: w76 -> [w96 w99]
          tunnel: [w95 w98] -> w75
          frame False {
            n22 = Build Array(w96, w97) -> (w95:dbl[][])
          }
          frame True {
            n23 = Build Array(w100, w99) -> (w98:dbl[][])
          }
        }
        "default module position on stave" <- w75
        n24 = Build Array(24.3 ("y"), 231.4 ("y"), 0.0 ("element"), -0.05 ("element")) -> ()  [unwired: 1 out]
        n25 = Build Array(0.0 ("element"), 238.0 ("element"), 0.0 ("element"), 0.0 ("element")) -> (w59:dbl[])
        n26 = Add(x=w57, y=w59) -> (x+y=w58:dbl[])
        n27 = Build Array(w57, w58) -> (w56:dbl[][])
        n28 = for {
          N: 2 -> [_]
          tunnel: w69 -> [w94]
          tunnel: [w94] -> w67 mode=indexing
          tunnel: w68 -> [w93]
          tunnel: [w93] -> w66 mode=indexing
        }
        n29 = Index Array(array=w65, index=3) -> (element=w73:dbl)
        n30 = for {
          tunnel: w75 -> [w108] mode=indexing
          tunnel: w73 -> [w102]
          tunnel: w57 -> [w107]
          tunnel: [w105] -> _ mode=indexing
          (unwired) 0 ("index")
          n31 = Multiply(x=w102, y=-1.0) -> (x*y=w103:dbl)
          n32 = Index Array(array=w108) -> (element=w111:dbl)  [unwired: 1 in]
          n33 = Index Array(array=w108, index=1) -> (element=w110:dbl)
          n34 = call-poly <vilib>:"2D Cartesian Coordinate Rotation.vi"("theta"=w103, "y"=w110, "x"=w111) -> ("y out"=w113:dbl, "x out"=w112:dbl)  [unwired: 6 in, 1 out]
          n35 = Build Array(w112, w113, 0.0 ("element"), 0.0 ("element")) -> (w106:dbl[])
          n36 = Add(x=w106, y=w107) -> (x+y=w105:dbl[])
        }
      }
      event "Measure HDI": Value Change {
        (unwired) "HDI alignment in progress ..." ("String")
        n37 = event-data() -> ()  [unwired: 1 in, 6 out]
        n38 = for {
          N: w116 -> [_]
          tunnel: w127 -> [w160]
          shift-right: [w149] -> w129
          shift-left: w130 -> [w158]
          tunnel: w128 -> [w159]
          tunnel: [w192] -> w120 mode=indexing
          tunnel: [w191] -> w122 mode=indexing
          tunnel: [w150] -> w121 mode=indexing
          tunnel: [w131] -> w115 mode=indexing
          (unwired) "ideal delta Y between \n2 fiducial marks"
          (unwired) "ideal delta X between 2 fiducial marks"
          # "1"
          # "3"
          n39 = call "Joystick and Camera SHIH VPC- external Connection.vi"("Motion in"=w158, "XYZTheta"=w159, "Measurement Point"="Measure Top-Left of HDI") -> ("Motion out"=w172:refnum<class "Motion.lvclass">, "Sum"=w135:dbl[])  [unwired: 4 in, 2 out]
          n40 = Add(x=w160, y=w135) -> (x+y=w142:dbl[])
          n41 = Index Array(array=w135, index=0) -> (element=w163:dbl)
          n42 = Array Subset(array=w142, index=0, length=2) -> (w175:dbl[])
          n43 = Replace Array Subset(array=w175, new element=w163, index=0) -> (w173:dbl[])
          n44 = call-dynamic "XY Go.vi"("Speed"=100.0, "XY"=w173, "Motion in"=w172) -> ("Motion out"=w179:refnum<class "Motion.lvclass">)  [unwired: 7 in, 1 out]
          n45 = Build Array(24.3 ("y"), 231.4 ("y"), 0.0 ("element"), -0.05 ("element")) -> ()  [unwired: 1 out]
          n46 = call "Joystick and Camera SHIH VPC- external Connection.vi"("Motion in"=w179, "Measurement Point"="Measure Bottom-Left of HDI", "Inital GO"=FALSE) -> ("Motion out"=w171:refnum<class "Motion.lvclass">, "Sum"=w134:dbl[])  [unwired: 4 in, 2 out]
          n47 = Array Subset(array=w142, index=0, length=2) -> (w185:dbl[])
          n48 = Subtract(x=w134, y=w135) -> (x-y=w170:dbl[])
          n49 = call-dynamic "XY Go.vi"("Speed"=100.0, "XY"=w185, "Motion in"=w171) -> ("Motion out"=w189:refnum<class "Motion.lvclass">)  [unwired: 7 in, 1 out]
          n50 = call "XY_to_Rotation_RPHI.vi"("X-Y"=w170) -> ("r-phi"=w166:dbl[])
          n51 = call "Joystick and Camera SHIH VPC- external Connection.vi"("Motion in"=w189, "Measurement Point"="Measure Bottom-Righ of HDI", "Inital GO"=FALSE) -> ("Motion out"=w147:refnum<class "Motion.lvclass">, "Sum"=w133:dbl[])  [unwired: 4 in, 2 out]
          n52 = Subtract(x=w133, y=w135) -> (x-y=w156:dbl[])
          n53 = Array Subset(array=w142, index=0, length=2) -> (w138:dbl[])
          n54 = Index Array(array=w135, index=1) -> (element=w139:dbl)
          n55 = Index Array(array=w166, index=1) -> (element=w161:dbl)
          n56 = Replace Array Subset(array=w138, new element=w139, index=1) -> (w137:dbl[])
          n57 = call-dynamic "XY Go.vi"("Speed"=100.0, "XY"=w137, "Motion in"=w147) -> ("Motion out"=w146:refnum<class "Motion.lvclass">)  [unwired: 7 in, 1 out]
          n58 = Multiply(x=w161, y=-1.0) -> (x*y=w154:dbl)
          n59 = Replace Array Subset(array=w156, new element=w154, index=3) -> (w191:dbl[])
          n60 = call "Joystick and Camera SHIH VPC- external Connection.vi"("Motion in"=w146, "Measurement Point"="Measure Top-right of HDI", "Inital GO"=FALSE) -> ("Motion out"=w149:refnum<class "Motion.lvclass">, "Sum"=w132:dbl[])  [unwired: 4 in, 2 out]
          n61 = Replace Array Subset(array=w135, new element=w154, index=3) -> (w192:dbl[])
          n62 = Add(x=w133, y=w135) -> (x+y=w194:dbl[])
          n63 = Divide(x=w194, y=2.0) -> (x/y=w153:dbl[])
          n64 = Build Array(w135, w134, w133, w132) -> (w131:dbl[][])
          n65 = Replace Array Subset(array=w153, new element=w154, index=3) -> (w151:dbl[])
          n66 = Subtract(x=w151, y=dbl[] [0.4, 0.4, 0.0, 0.0]) -> (x-y=w150:dbl[])
        }
        "North" <- w115
        "South" <- w115
      }
      event "Stop": Value Change {
        n67 = event-data() -> ()  [unwired: 1 in, 6 out]
        n68 = call "XYZTheta Go.vi"("XYZTheta In"=dbl[] [625.0, 625.0, 0.0, 0.01], "Motion in"=w211) -> ("Motion out"=w209:refnum<class "Motion.lvclass">)  [unwired: 7 in, 2 out]
      }
      event "Align Stave": Value Change {
        # "center of lower module"
        # "center of upper module"
        # "Default stave dimension\namong mounting holes"
        # "Measure 2 module positions on stave"
        n69 = event-data() -> ()  [unwired: 1 in, 6 out]
        n70 = Build Array(34.0 ("element"), 470.0 ("element"), 0.0 ("element"), 0.0 ("element")) -> ()  [unwired: 1 out]
        n71 = for {
          N: 1 -> [_]
          tunnel: w242 -> [w259]
          shift-right: [w269] -> w241
          shift-left: w244 -> [w270]
          tunnel: w243 -> [w271]
          tunnel: [w264] -> w217
          tunnel: [w262] -> w227
          (unwired) "ideal delta Y between \n2 fiducial marks"
          (unwired) "ideal delta X between 2 fiducial marks"
          n72 = call "Joystick and Camera SHIH VPC- external Connection.vi"("Motion in"=w270, "XYZTheta"=w271, "Measurement Point"="Measure Top-Left of stave") -> ("Motion out"=w253:refnum<class "Motion.lvclass">, "Sum"=w255:dbl[])  [unwired: 4 in, 2 out]
          n73 = Replace Array Subset(array=w259, new element=0.0 ("new element/subarray"), index=0) -> (w256:dbl[])
          n74 = Add(x=w255, y=w256) -> (x+y=w254:dbl[])
          n75 = call "Joystick and Camera SHIH VPC- external Connection.vi"("Motion in"=w253, "XYZTheta"=w254, "Measurement Point"="Measure Bottom-Left of stave", "Inital GO"=TRUE) -> ("Motion out"=w261:refnum<class "Motion.lvclass">, "Sum"=w274:dbl[])  [unwired: 3 in, 2 out]
          n76 = Build Array(24.3 ("y"), 231.4 ("y"), 0.0 ("element"), -0.05 ("element")) -> ()  [unwired: 1 out]
          n77 = Add(x=w259, y=w255) -> (x+y=w260:dbl[])
          n78 = Subtract(x=w274, y=w255) -> (x-y=w280:dbl[])
          n79 = call "XY_to_Rotation_RPHI.vi"("X-Y"=w280) -> ("r-phi"=w276:dbl[])
          n80 = Index Array(array=w276, index=1) -> (element=w272:dbl)
          n81 = call "Joystick and Camera SHIH VPC- external Connection.vi"("Motion in"=w261, "XYZTheta"=w260, "Measurement Point"="Measure Bottom-Righ of stave", "Inital GO"=TRUE) -> ("Motion out"=w269:refnum<class "Motion.lvclass">, "Sum"=w266:dbl[])  [unwired: 3 in, 2 out]
          n82 = Subtract(x=w266, y=w255) -> (x-y=w267:dbl[])
          n83 = Multiply(x=w272, y=-1.0) -> (x*y=w262:dbl)
          n84 = Replace Array Subset(array=w267, new element=w262, index=3) -> (→"measured stave size":dbl[])
          n85 = Replace Array Subset(array=w255, new element=w262, index=3) -> (w264:dbl[])
          n86 = Add(x=w266, y=w255) -> (x+y=w288:dbl[])
          n87 = Divide(x=w288, y=2.0) -> (x/y=→"Center of module on stave":dbl[])
        }
        n88 = Build Array(0.0 ("element"), 238.0 ("element"), 0.0 ("element"), 0.0 ("element")) -> (w218:dbl[])
        n89 = Add(x=w217, y=w218) -> (x+y=w216:dbl[])
        n90 = Build Array(w217, w216) -> (w215:dbl[][])
        n91 = Build Array(17.0 ("element"), 411.0 ("element"), 0.0 ("element"), 0.0 ("element")) -> (w229:dbl[])
        n92 = Build Array(17.0 ("element"), 60.9 ("element"), 0.0 ("element"), 0.0 ("element")) -> (w230:dbl[])
        n93 = case shown="True" w225 {
          tunnel: w230 -> [w307 w310]
          tunnel: w229 -> [w306 w309]
          tunnel: [w305 w308] -> w228
          frame False {
            n94 = Build Array(w306, w307) -> (w305:dbl[][])
          }
          frame True {
            n95 = Build Array(w310, w309) -> (w308:dbl[][])
          }
        }
        n96 = for {
          tunnel: w228 -> [w298] mode=indexing
          tunnel: w227 -> [w293]
          tunnel: w217 -> [w297]
          tunnel: [w295] -> w224 mode=indexing
          n97 = Multiply(x=w293, y=-1.0) -> (x*y=w292:dbl)
          n98 = Index Array(array=w298, index=0) -> (element=w301:dbl)
          n99 = Index Array(array=w298, index=1) -> (element=w300:dbl)
          n100 = call-poly <vilib>:"2D Cartesian Coordinate Rotation.vi"("theta"=w292, "y"=w300, "x"=w301) -> ("y out"=w303:dbl, "x out"=w302:dbl)  [unwired: 6 in, 1 out]
          n101 = Build Array(w302, w303, 0.0 ("element"), 0.0 ("element")) -> (w296:dbl[])
          n102 = Add(x=w296, y=w297) -> (x+y=w295:dbl[])
        }
      }
      event "Align Stave in detail": Value Change {
        # "center of lower module"
        # "center of upper module"
        # "Default stave dimension\namong mounting holes"
        # "Measure 2 module positions on stave"
        n103 = event-data() -> ()  [unwired: 1 in, 6 out]
        n104 = Build Array(34.0 ("element"), 470.0 ("element"), 0.0 ("element"), 0.0 ("element")) -> ()  [unwired: 1 out]
        n105 = for {
          N: 1 -> [_]
          tunnel: w341 -> [w358]
          shift-right: [w368] -> w340
          shift-left: w343 -> [w369]
          tunnel: w342 -> [w370]
          tunnel: [w363] -> w316
          tunnel: [w361] -> w326
          (unwired) "ideal delta Y between \n2 fiducial marks"
          (unwired) "ideal delta X between 2 fiducial marks"
          n106 = call "Joystick and Camera SHIH V5- external Connection.vi"("Motion in"=w369, "XYZTheta"=w370, "Measurement Point"="Measure Top-Left of stave") -> ("final out"=w354:dbl[], "Motion out"=w352:refnum<class "Motion.lvclass">)  [unwired: 5 in, 1 out]
          n107 = Replace Array Subset(array=w358, new element=0.0 ("new element/subarray"), index=0) -> (w355:dbl[])
          n108 = Add(x=w354, y=w355) -> (x+y=w353:dbl[])
          n109 = call "Joystick and Camera SHIH V5- external Connection.vi"("Motion in"=w352, "XYZTheta"=w353, "Measurement Point"="Measure Bottom-Left of stave", "Inital GO"=TRUE) -> ("final out"=w373:dbl[], "Motion out"=w360:refnum<class "Motion.lvclass">)  [unwired: 4 in, 1 out]
          n110 = Build Array(24.3 ("y"), 231.4 ("y"), 0.0 ("element"), -0.05 ("element")) -> ()  [unwired: 1 out]
          n111 = Add(x=w358, y=w354) -> (x+y=w359:dbl[])
          n112 = Subtract(x=w373, y=w354) -> (x-y=w379:dbl[])
          n113 = call "XY_to_Rotation_RPHI.vi"("X-Y"=w379) -> ("r-phi"=w375:dbl[])
          n114 = Index Array(array=w375, index=1) -> (element=w371:dbl)
          n115 = call "Joystick and Camera SHIH V5- external Connection.vi"("Motion in"=w360, "XYZTheta"=w359, "Measurement Point"="Measure Bottom-Righ of stave", "Inital GO"=TRUE) -> ("final out"=w365:dbl[], "Motion out"=w368:refnum<class "Motion.lvclass">)  [unwired: 4 in, 1 out]
          n116 = Subtract(x=w365, y=w354) -> (x-y=w366:dbl[])
          n117 = Multiply(x=w371, y=-1.0) -> (x*y=w361:dbl)
          n118 = Replace Array Subset(array=w366, new element=w361, index=3) -> (→"FROM Detail !! measured stave size":dbl[])
          n119 = Replace Array Subset(array=w354, new element=w361, index=3) -> (w363:dbl[])
          n120 = Add(x=w365, y=w354) -> (x+y=w387:dbl[])
          n121 = Divide(x=w387, y=2.0) -> (x/y=→"FROM Detail !!! Center of module on stave":dbl[])
        }
        n122 = Build Array(0.0 ("element"), 238.0 ("element"), 0.0 ("element"), 0.0 ("element")) -> (w317:dbl[])
        n123 = Add(x=w316, y=w317) -> (x+y=w315:dbl[])
        n124 = Build Array(w316, w315) -> (w314:dbl[][])
        n125 = Build Array(17.0 ("element"), 411.0 ("element"), 0.0 ("element"), 0.0 ("element")) -> (w328:dbl[])
        n126 = Build Array(17.0 ("element"), 60.9 ("element"), 0.0 ("element"), 0.0 ("element")) -> (w329:dbl[])
        n127 = case shown="True" w324 {
          tunnel: w329 -> [w406 w409]
          tunnel: w328 -> [w405 w408]
          tunnel: [w404 w407] -> w327
          frame False {
            n128 = Build Array(w405, w406) -> (w404:dbl[][])
          }
          frame True {
            n129 = Build Array(w409, w408) -> (w407:dbl[][])
          }
        }
        n130 = for {
          tunnel: w327 -> [w397] mode=indexing
          tunnel: w326 -> [w392]
          tunnel: w316 -> [w396]
          tunnel: [w394] -> w323 mode=indexing
          n131 = Multiply(x=w392, y=-1.0) -> (x*y=w391:dbl)
          n132 = Index Array(array=w397, index=0) -> (element=w400:dbl)
          n133 = Index Array(array=w397, index=1) -> (element=w399:dbl)
          n134 = call-poly <vilib>:"2D Cartesian Coordinate Rotation.vi"("theta"=w391, "y"=w399, "x"=w400) -> ("y out"=w402:dbl, "x out"=w401:dbl)  [unwired: 6 in, 1 out]
          n135 = Build Array(w401, w402, 0.0 ("element"), 0.0 ("element")) -> (w395:dbl[])
          n136 = Add(x=w395, y=w396) -> (x+y=w394:dbl[])
        }
      }
      event "Bless from OGP": Value Change {
        # "center of upper module"
        # "center of lower module"
        # "center of upper module"
        # "NL line with correct rotation"
        # "Default stave dimension\namong mounting holes"
        # "Measure 2 module positions on stave"
        n137 = event-data() -> ()  [unwired: 1 in, 6 out]
        n138 = Build Array(34.0 ("element"), 470.0 ("element"), 0.0 ("element"), 0.0 ("element")) -> ()  [unwired: 1 out]
        n139 = for {
          N: 1 -> [_]
          tunnel: w461 -> [_]
          shift-right: [w521] -> w460
          shift-left: w444 -> [w534]
          tunnel: w446 -> [_]
          tunnel: [w513] -> w449
          tunnel: [w516] -> w457
          tunnel: w445 -> [w523]
          tunnel: [w499] -> w432
          (unwired) FALSE ("Inital GO")
          (unwired) "ideal delta Y between \n2 fiducial marks"
          (unwired) "ideal delta X between 2 fiducial marks"
          # "after NL"
          # "after SL"
          # "NL line"
          # "rotation"
          n140 = call "Joystick and Camera SHIH VPC- external Connection.vi"("Motion in"=w534, "XYZTheta"=dbl[] [576.333, 663.131, 70.7812, 0.010000094994154989] ("N chip"), "Measurement Point"="north chip", "Inital GO"=TRUE) -> ("Motion out"=w531:refnum<class "Motion.lvclass">, "Sum"=w511:dbl[])  [unwired: 3 in, 2 out]
          "N chip" <- w511
          n141 = call "Joystick and Camera SHIH VPC- external Connection.vi"("Motion in"=w531, "XYZTheta"=dbl[] [578.791, 1154.64, 70.5935, 0.010000670236950445] ("S chip"), "Measurement Point"="south chip", "Inital GO"=TRUE) -> ("Motion out"=w530:refnum<class "Motion.lvclass">, "Sum"=w512:dbl[])  [unwired: 3 in, 2 out]
          "S chip" <- w512
          n142 = Subtract(x=w512, y=w511) -> (x-y=w510:dbl[])
          n143 = Index Array(array=w510, index #1=0 ("index"), index #2=1 ("index")) -> (element #1=w507:dbl, element #2=w506:dbl)
          n144 = Square(x=w507) -> (x^2=w504:dbl)
          n145 = Square(x=w506) -> (x^2=w505:dbl)
          n146 = Add(x=w504, y=w505) -> (x+y=w503:dbl)
          n147 = call "Joystick and Camera SHIH VPC- external Connection.vi"("Motion in"=w530, "Measurement Point"="height of stave", "Inital GO"=FALSE) -> ("Motion out"=w521:refnum<class "Motion.lvclass">, "Sum"=w522:dbl[])  [unwired: 4 in, 2 out]
          n148 = call "O to G peek.vi"("height"=w522, "south chip"=w512, "north chip"=w511, "Input file"=w523) -> ("OGP length"=→"chip distance by OGP":dbl, "output BR"=w525:dbl[], "output BL"=w524:dbl[], "output TL"=w518:dbl[])  [unwired: 4 in]
          "after NL" <- w518
          "after SR" <- w525
          "after SL" <- w524
          n149 = Square Root(x=w503) -> (sqrt(x)=→"chip distance by gantry":dbl)
          n150 = Subtract(x=w525, y=w518) -> (x-y=w536:dbl[])
          n151 = Build Array(24.3 ("y"), 231.4 ("y"), 0.0 ("element"), -0.05 ("element")) -> ()  [unwired: 1 out]
          n152 = Subtract(x=w524, y=w518) -> (x-y=w542:dbl[])
          n153 = call "XY_to_Rotation_RPHI.vi"("X-Y"=w542) -> ("r-phi"=w541:dbl[])
          n154 = Index Array(array=w541, index=1) -> (element=w538:dbl)
          n155 = Multiply(x=w538, y=-1.0) -> (x*y=w516:dbl)
          n156 = Replace Array Subset(array=w536, new element=w516, index=3) -> (→"bless from OGP !! measured stave size":dbl[])
          n157 = Replace Array Subset(array=w518, new element=w516, index=3) -> (w514:dbl[])
          n158 = Add(x=w525, y=w518) -> (x+y=w548:dbl[])
          n159 = Divide(x=w548, y=2.0) -> (x/y=w500:dbl[])
          n160 = Add(x=w514, y=dbl[] [0.0, 10.0, 0.0, 0.0]) -> (x+y=w513:dbl[])
          n161 = Replace Array Subset(array=w500, new element=w516, index=3) -> (w499:dbl[])
          "bless from OGP !!! Center of  stave" <- w499
        }
        n162 = Build Array(0.0 ("element"), 238.0 ("element"), 0.0 ("element"), 0.0 ("element")) -> (w450:dbl[])
        n163 = Add(x=w449, y=w450) -> (x+y=w448:dbl[])
        n164 = Build Array(w449, w448) -> (w447:dbl[][])
        n165 = Build Array(0.0 ("element"), 116.65 ("element"), 0.0 ("element"), 0.0 ("element")) -> (w433:dbl[])
        n166 = Build Array(0.0 ("element"), -116.65 ("element"), 0.0 ("element"), 0.0 ("element")) -> (w434:dbl[])
        n167 = Build Array(0.0 ("element"), 116.65 ("element"), 0.0 ("element"), 0.0 ("element")) -> (w415:dbl[])
        n168 = Build Array(0.0 ("element"), -116.65 ("element"), 0.0 ("element"), 0.0 ("element")) -> (w416:dbl[])
        n169 = case shown="False" w414 {
          tunnel: w434 -> [w495 w498]
          tunnel: w433 -> [w494 w497]
          tunnel: [w493 w496] -> w431
          frame False {
            n170 = Build Array(w494, w495) -> (w493:dbl[][])
          }
          frame True {
            n171 = Build Array(w498, w497) -> (w496:dbl[][])
          }
        }
        n172 = case shown="True" w414 {
          tunnel: w416 -> [w472 w475]
          tunnel: w415 -> [w471 w474]
          tunnel: [w470 w473] -> w413
          frame False {
            n173 = Build Array(w471, w472) -> (w470:dbl[][])
          }
          frame True {
            n174 = Build Array(w475, w474) -> (w473:dbl[][])
          }
        }
        n175 = for {
          tunnel: w431 -> [w569] mode=indexing
          tunnel: w457 -> [w566]
          tunnel: [w568] -> w443 mode=indexing
          tunnel: w432 -> [w551]
          tunnel: [w563] -> w430 mode=indexing
          tunnel: w413 -> [w554] mode=indexing
          tunnel: [w550] -> w412 mode=indexing
          n176 = Multiply(x=w566, y=-1.0) -> (x*y=w553:dbl)
          n177 = Index Array(array=w569, index=0) -> (element=w572:dbl)
          n178 = Index Array(array=w569, index=1) -> (element=w571:dbl)
          n179 = Index Array(array=w554, index=0) -> (element=w559:dbl)
          n180 = Index Array(array=w554, index=1) -> (element=w558:dbl)
          n181 = call-poly <vilib>:"2D Cartesian Coordinate Rotation.vi"("theta"=w553, "y"=w571, "x"=w572) -> ("y out"=w574:dbl, "x out"=w573:dbl)  [unwired: 6 in, 1 out]
          n182 = call-poly <vilib>:"2D Cartesian Coordinate Rotation.vi"("theta"=w553, "y"=w558, "x"=w559) -> ("y out"=w561:dbl, "x out"=w560:dbl)  [unwired: 6 in, 1 out]
          n183 = Build Array(w573, w574, 0.0 ("element"), 0.0 ("element")) -> (w563:dbl[])
          n184 = Build Array(w560, w561, 0.0 ("element"), 0.0 ("element")) -> (w552:dbl[])
          n185 = Add(x=w552, y=w551) -> (x+y=w550:dbl[])
          n186 = Add(x=w563, y=w551) -> (x+y=w568:dbl[])
        }
        "CT HPoS" <- w430
        "HDI center positions" <- w412
        n187 = Add(x=w443, y=w429) -> (x+y=w428:dbl[][])
        n188 = call-poly <vilib>:"Write Delimited Spreadsheet.vi"("file path (dialog if empty)"=path "D:/INTT/V1/Assembly Data/ladder assembly/2line_switch.txt", "format (%.3f)"="%.10f", "2D data"=w428) -> ()  [unwired: 11 in, 2 out]
        n189 = disable-structure shown="Disabled" {
          disable-tunnel: w414 -> [w476 _]
          frame Disabled {
            # "center of lower module"
            # "center of upper module"
            n190 = Build Array(17.0 ("element"), 60.9 ("element"), 0.0 ("element"), 0.0 ("element")) -> (w478:dbl[])
            n191 = Build Array(17.0 ("element"), 411.0 ("element"), 0.0 ("element"), 0.0 ("element")) -> (w477:dbl[])
            n192 = case shown="True" w476 {
              tunnel: w478 -> [w489 w492]
              tunnel: w477 -> [w488 w491]
              tunnel: [w487 w490] -> _
              frame False {
                n193 = Build Array(w488, w489) -> (w487:dbl[][])
              }
              frame True {
                n194 = Build Array(w492, w491) -> (w490:dbl[][])
              }
            }
          }
          frame Enabled {
          }
        }
      }
      event "txt switch": Value Change {
        n195 = event-data() -> ()  [unwired: 1 in, 6 out]
        n196 = flat-sequence {
          tunnel: [w599] -> w593
          tunnel: w583 -> [w595]
          tunnel: [w595] -> w582
          tunnel: w580 -> [w594]
          tunnel: [w594] -> w579
          tunnel: w593 -> [w617]
          tunnel: [w615] -> w581
          tunnel: w582 -> [w615]
          tunnel: [w614] -> w578
          tunnel: w579 -> [w614]
          frame #0 {
            n197 = call-poly <vilib>:"Read Delimited Spreadsheet.vi"("file path (dialog if empty)"=path "D:/INTT/V1/Assembly Data/ladder assembly/2line_switch.txt" ("file path (dialog if empty) 3"), "format (%.3f)"="%.10f") -> ("all rows"=w600:dbl[][])  [unwired: 8 in, 5 out]
            n198 = Array Subset(array=w600, index (row)=0 ("index"), length (row)=1 ("length"), index (col)=0 ("index"), length (col)=4 ("length")) -> (w610:dbl[][])
            n199 = Reshape Array(w610, 4 ("dimension size")) -> (w597:dbl[])
            n200 = Array Subset(array=w600, index (row)=1 ("index"), length (row)=1 ("length"), index (col)=0 ("index"), length (col)=4 ("length")) -> (w604:dbl[][])
            n201 = Reshape Array(w604, 4 ("dimension size")) -> (w598:dbl[])
            n202 = Build Array(w598, w597) -> (w599:dbl[][])
          }
          frame #1 {
            n203 = call-poly <vilib>:"Write Delimited Spreadsheet.vi"("file path (dialog if empty)"=path "D:/INTT/V1/Assembly Data/ladder assembly/2line_switch.txt" ("file path (dialog if empty) 4"), "format (%.3f)"="%.10f", "2D data"=w617) -> ()  [unwired: 11 in, 2 out]
          }
        }
      }
      event "Measure Pickup Tools": Value Change {
        (unwired) "Measuring Pickup Tools" ("String")
        n204 = event-data() -> ()  [unwired: 1 in, 6 out]
        n205 = for {
          N: w621 -> [_]
          tunnel: [w657] -> w632 mode=indexing
          tunnel: w633 -> [w661]
          tunnel: [w643] -> w631
          tunnel: w630 -> [w642] mode=indexing
          # "Default size and\norientation"
          n206 = call "Joystick and Camera SHIH VPC- external Connection.vi"("Motion in"=w661, "XYZTheta"=w642, "Measurement Point"="PickUp tool Top") -> ("Motion out"=w637:refnum<class "Motion.lvclass">, "Sum"=w660:dbl[])  [unwired: 4 in, 2 out]
          n207 = Build Array(0.0 ("element"), 29.94 ("element"), 0.0 ("element"), 0.0 ("element")) -> (w648:dbl[])
          n208 = Add(x=w660, y=w648) -> (x+y=w634:dbl[])
          n209 = Array Subset(array=w634, index=0, length=2) -> (w635:dbl[])
          n210 = call-dynamic "XY Go.vi"("Speed"=20.0, "XY"=w635, "Motion in"=w637) -> ("Motion out"=w636:refnum<class "Motion.lvclass">)  [unwired: 7 in, 1 out]
          n211 = call "Joystick and Camera SHIH VPC- external Connection.vi"("Motion in"=w636, "Measurement Point"="PickUp tool Bottom", "Inital GO"=FALSE) -> ("Motion out"=w643:refnum<class "Motion.lvclass">, "Sum"=w659:dbl[])  [unwired: 4 in, 2 out]
          n212 = Add(x=w660, y=w659) -> (x+y=w666:dbl[])
          n213 = Subtract(x=w659, y=w660) -> (x-y=w658:dbl[])
          n214 = Divide(x=w666, y=2.0) -> (x/y=w663:dbl[])
          n215 = call "XYtoRPHI.vi"("X-Y"=w658) -> ("r-phi"=w664:dbl[])
          n216 = Index Array(array=w664, index=1) -> (element=w652:dbl)
          n217 = Absolute Value(x=w652) -> (abs(x)=w655:dbl)
          n218 = Sign(1:w652) -> (0:w653:dbl)
          n219 = Subtract(x=w655, y=1.5707963267948966) -> (x-y=w654:dbl)
          n220 = Multiply(x=w653, y=w654) -> (x*y=w651:dbl)
          n221 = Replace Array Subset(array=w663, new element=w651, index=3) -> (w657:dbl[])
          "PickupTool \nCenterPosition" <- w657
        }
      }
      event "Deposit Glue": Value Change {
        (unwired) 20.0 ("Speed")
        # "purple"
        # "dark green"
        # "green"
        # "CF height"
        # "surface z offset"
        # "two sensor, Sensor B then A"
        # "Unmount syringe"
        # "first needle park position\nneedle gap on Z value : 0.5 mm"
        # "Syringe-camera offset"
        n222 = event-data() -> ()  [unwired: 1 in, 6 out]
        n223 = call-poly <vilib>:"Read Delimited Spreadsheet.vi"("file path (dialog if empty)"=path "D:/INTT/V1/Assembly Data/Tool Offsets/Dispense Tip Offset.txt", "number of rows (all:-1)"=-1) -> ("first row"=w722:dbl[])  [unwired: 8 in, 5 out]
        n224 = Add(x=14.2 ("element"), y=w686) -> (x+y=w680:dbl)
        n225 = Index Array(array=w722, index #1=0 ("index"), index #2=1 ("index")) -> (element #1=w717:dbl, element #2=w715:dbl)
        n226 = Build Array(w717, w715, 0.0 ("element"), 0.0 ("element")) -> (w706:dbl[])
        n227 = Array Subset(array=w676, index (row)=0, length (row)=1 ("length")) -> (w687:dbl[][])  [unwired: 2 in]
        n228 = Reshape Array(w687, 4 ("dimension size")) -> (w682:dbl[])
        n229 = Index Array(array=w682, index=2) -> (element=w677:dbl)
        n230 = Add(x=w677, y=w680) -> (x+y=w679:dbl)
        n231 = Build Array(427.051, 722.276, w679, 0.0 ("element")) -> (w678:dbl[])
        "Needle parking position" <- w678
        n232 = call "XYZTheta Go.vi"("XYZTheta In"=w678, "Motion in"=w709) -> ("error out"=w714:errorcluster, "Motion out"=w708:refnum<class "Motion.lvclass">)  [unwired: 7 in, 1 out]
        n233 = call "Display Message to User"("error in (no error)"=w714) -> ("error out"=w710:errorcluster)  [unwired: 9 in, 1 out]
        n234 = case shown="False" w684 {
          tunnel: w676 -> [w730 w739]
          tunnel: [w727 w739] -> w683
          frame False {
            n235 = Array Subset(array=w730, index (row)=1 ("index"), length (row)=1 ("length")) -> (w731:dbl[][])  [unwired: 2 in]
            n236 = Array Subset(array=w730, index (row)=0 ("index"), length (row)=1 ("length")) -> (w734:dbl[][])  [unwired: 2 in]
            n237 = Reshape Array(w734, 4 ("dimension size")) -> (w729:dbl[])
            n238 = Reshape Array(w731, 4 ("dimension size")) -> (w728:dbl[])
            n239 = Build Array(w728, w729) -> (w727:dbl[][])
          }
          frame True {
          }
        }
        n240 = call-dynamic "Z Go.vi"("error in (no error)"=w710, "Speed"=20.0, "Position"=0.0, "Motion in"=w708) -> ("error out"=w707:errorcluster, "Motion out"=w671:refnum<class "Motion.lvclass">)  [unwired: 6 in]
        n241 = Add(x=w677, y=-2.5) -> ()  [unwired: 1 out]
        n242 = call "Display Message to User2"("error in (no error)"=w707) -> ("error out"=w670:errorcluster)  [unwired: 9 in, 1 out]
        n243 = call-dynamic "Connect.vi"("Ultimus V in"=refnum<class "Ultimus V2.lvclass"> refnum ("Ultimus V2.lvclass")) -> ("Ultimus V out"=w705:refnum<class "Ultimus V2.lvclass">)  [unwired: 9 in, 1 out]
        n244 = for {
          N: w673 -> [_]
          tunnel: w705 -> [w749]
          tunnel: w706 -> [w744]
          tunnel: w683 -> [_] mode=indexing
          tunnel: [w747] -> w694
          tunnel: [w746] -> w693
          tunnel: w670 -> [w742]
          tunnel: w685 -> [_]
          tunnel: [w745] -> w674
          tunnel: w668 -> [_] mode=indexing
          tunnel: w668 -> [w748] mode=indexing
          tunnel: w671 -> [w743]
          tunnel: w669 -> [w740]
          i -> [w741]
          (unwired) dbl[][] [[3.038, 0.63], [7.0, 0.0], [0.0, -206.0], [-7.0, 0.0]] ("distances")
          (unwired) dbl[] [-1.774, -0.587, 0.0, 0.0] ("distances")
          n245 = for {
            N: 4 -> [_]
            tunnel: w743 -> [w787]
            tunnel: w749 -> [w791]
            tunnel: w742 -> [w785]
            tunnel: w748 -> [w764] mode=indexing
            tunnel: [w784] -> w747
            tunnel: [w783] -> w746
            tunnel: [w771] -> w745
            tunnel: w744 -> [w779]
            tunnel: w741 -> [w758]
            tunnel: w740 -> [w752]
            i -> [w770]
            n246 = Multiply(x=w758, y=4) -> (x*y=w755:i32)
            n247 = Increment(x=w770) -> (x+1=w756:i32)
            n248 = Add(x=w755, y=w756) -> (x+y=w754:i32)
            "corner index" <- w754
            n249 = Index Array(array=w764, index=2) -> (element=w762:dbl)
            n250 = case shown="1, Default" w754 {
              tunnel: [dbl[] [-2.158, -0.64, 0.0, 0.0] ("distances") dbl[] [-2.196, -0.521, 0.0, 0.0] ("distances") dbl[] [1.449, -0.438, 0.0, 0.0] ("distances") dbl[] [1.217, -0.563, 0.0, 0.0] ("distances") dbl[] [-2.198, -0.263, 0.0, 0.0] ("distances") dbl[] [-2.02, -0.187, 0.0, 0.0] ("distances") dbl[] [1.449, -0.186, 0.0, 0.0] ("distances") dbl[] [1.381, -0.3, 0.0, 0.0] ("distances")] -> w776
              tunnel: [dbl[][] [[3.552, 0.733], [7.0, 0.0], [0.0, -206.0], [-7.0, 0.0]] ("distances") dbl[][] [[3.557, -0.3], [7.0, 0.0], [0.0, -206.0], [-7.0, 0.0]] ("distances") dbl[][] [[-3.736, -0.48], [7.0, 0.0], [0.0, -206.0], [-7.0, 0.0]] ("distances") dbl[][] [[-3.512, 0.563], [7.0, 0.0], [0.0, -206.0], [-7.0, 0.0]] ("distances") dbl[][] [[3.616, 0.287], [7.0, 0.0], [0.0, -206.0], [-7.0, 0.0]] ("distances") dbl[][] [[3.453, -0.694], [7.0, 0.0], [0.0, -206.0], [-7.0, 0.0]] ("distances") dbl[][] [[-3.647, -0.637], [7.0, 0.0], [0.0, -206.0], [-7.0, 0.0]] ("distances") dbl[][] [[-3.66, 0.357], [7.0, 0.0], [0.0, -206.0], [-7.0, 0.0]] ("distances")] -> w775
              frame 1, Default {
              }
              frame 2 {
              }
              frame 3 {
              }
              frame 4 {
                # "Y"
                # "X"
              }
              frame 5 {
              }
              frame 6 {
              }
              frame 7 {
              }
              frame 8 {
              }
            }
            n251 = Add(x=w776, y=w764) -> (x+y=w778:dbl[])
            n252 = Add(x=w779, y=w778) -> (x+y=w777:dbl[])
            n253 = Array Subset(array=w777, index=0, length=2) -> (w780:dbl[])
            "x+y" <- w780
            n254 = call-dynamic "XY Go.vi"("error in (no error)"=w785, "Speed"=80.0, "XY"=w780, "Motion in"=w787) -> ("error out"=w767:errorcluster, "Motion out"=w769:refnum<class "Motion.lvclass">)  [unwired: 6 in]
            n255 = Subtract(x=5.5818 ("y"), y=w752) -> (x-y=w751:dbl)
            n256 = Add(x=w762, y=w751) -> (x+y=w759:dbl)
            n257 = call-dynamic "Z Go.vi"("error in (no error)"=w767, "Speed"=5.0, "Position"=w759, "Motion in"=w769) -> ("error out"=w766:errorcluster, "Motion out"=w768:refnum<class "Motion.lvclass">)  [unwired: 6 in]
            n258 = flat-sequence {
              tunnel: w791 -> [w831]
              tunnel: [w831] -> w792
              tunnel: w792 -> [w834]
              tunnel: [w834] -> w790
              tunnel: [w833] -> w788
              tunnel: [w832] -> w789
              frame #0 {
              }
              frame #1 {
                n259 = call "air pressure setting.vi"() -> ("air pressure indecator"=w833:i32, "deposit speed 2"=w832:dbl)
              }
            }
            n260 = flat-sequence {
              tunnel: w766 -> [w801]
              tunnel: w768 -> [w800]
              tunnel: [w797] -> w761
              tunnel: [w798] -> w760
              tunnel: w759 -> [w794]
              tunnel: w790 -> [w810]
              tunnel: w789 -> [w809]
              tunnel: w788 -> [w808]
              tunnel: w775 -> [w803]
              tunnel: [w805] -> w774
              tunnel: [w804] -> w773
              tunnel: [w802] -> w772
              tunnel: w761 -> [w806]
              tunnel: w760 -> [w802]
              tunnel: [w813] -> w783
              tunnel: [w814] -> w784
              tunnel: w774 -> [w814]
              tunnel: w773 -> [w813]
              tunnel: w772 -> [w812]
              tunnel: [w811] -> w771
              frame #0 {
                n261 = call "?"("error in (no error)"=w801) -> ("error out"=w799:errorcluster)  [unwired: 9 in, 1 out]
                n262 = Subtract(x=w794, y=3.0) -> (x-y=w793:dbl)
                n263 = call-dynamic "Z Go.vi"("error in (no error)"=w799, "Speed"=5.0, "Position"=w793, "Motion in"=w800) -> ("error out"=w798:errorcluster, "Motion out"=w797:refnum<class "Motion.lvclass">)  [unwired: 6 in]
              }
              frame #1 {
                n264 = call "Muliti_XY_dispense_shih.vi"("Pressure"=w808, "Path count"=1, "Speed"=w809, "distances"=w803, "Ultimus V in"=w810, "Motion in"=w806) -> ("Ultimus V out"=w804:refnum<class "Ultimus V2.lvclass">, "Motion out"=w805:refnum<class "Motion.lvclass">)  [unwired: 4 in]
              }
              frame #2 {
                n265 = call "Time Delay5"("error in (no error)"=w812) -> ("error out"=w811:errorcluster)  [unwired: 10 in]
              }
            }
            "Array" <- w764
          }
        }
        n266 = call "XYZTheta Go.vi"("error in (no error)"=w674, "XYZTheta In"=dbl[] [500.0, 1000.0, 0.0, 0.1], "Motion in"=w694) -> ("error out"=w703:errorcluster, "Motion out"=w701:refnum<class "Motion.lvclass">)  [unwired: 6 in, 1 out]
        n267 = call "Display Message to User3"("error in (no error)"=w703) -> ()  [unwired: 9 in, 2 out]
        n268 = call-dynamic "Disconnect.vi"("Ultimus V in"=w693) -> ()  [unwired: 9 in, 1 out]
      }
      event "Needle Alignment": Value Change {
        (unwired) "Needle Alignment in progress ...." ("String")
        # "CF height"
        # "surface z offset"
        # "first needle park position\nneedle gap on Z value : 0.5 mm"
        # "Syringe-camera offset"
        n269 = event-data() -> ()  [unwired: 1 in, 6 out]
        n270 = Array Subset(array=w839, index (row)=0, length (row)=1 ("length")) -> (w842:dbl[][])  [unwired: 2 in]
        n271 = Reshape Array(w842, 4 ("dimension size")) -> (w841:dbl[])
        n272 = Index Array(array=w841, index=2) -> (element=w838:dbl)
        n273 = call-poly <vilib>:"Read Delimited Spreadsheet.vi"("file path (dialog if empty)"=path "D:/INTT/V1/Assembly Data/Tool Offsets/Dispense Tip Offset.txt", "number of rows (all:-1)"=-1) -> ("first row"=w889:dbl[])  [unwired: 8 in, 5 out]
        n274 = Index Array(array=w889, index #1=0 ("index"), index #2=1 ("index")) -> (element #1=w884:dbl, element #2=w883:dbl)
        n275 = Add(x=14.2 ("element"), y=w847) -> (x+y=w849:dbl)
        n276 = Add(x=w838, y=w849) -> (x+y=w848:dbl)
        n277 = Build Array(424.448, 1040.76, w848, 0.0 ("element")) -> (w846:dbl[])
        n278 = Build Array(w884, w883, 0.0 ("element"), 0.0 ("element")) -> (w858:dbl[])
        n279 = call "XYZTheta Go.vi"("XYZTheta In"=w846, "Motion in"=w873) -> ("error out"=w882:errorcluster, "XYZTheta Out"=w863:dbl[], "Motion out"=w872:refnum<class "Motion.lvclass">)  [unwired: 7 in]
        n280 = call "Display Message to User10"("error in (no error)"=w882) -> ("error out"=w879:errorcluster)  [unwired: 9 in, 1 out]
        n281 = call-dynamic "Z Go.vi"("error in (no error)"=w879, "Speed"=20.0, "Position"=0.0, "Motion in"=w872) -> ("Motion out"=w871:refnum<class "Motion.lvclass">)  [unwired: 6 in, 1 out]
        n282 = Replace Array Subset(array=w863, new element=0.0 ("new element/subarray"), index=2) -> (w860:dbl[])
        n283 = call "Joystick and Camera SHIH VPC- external Connection.vi"("Motion in"=w871, "XYZTheta"=w860, "Measurement Point"="Touch Needle on a surface") -> ("Motion out"=w869:refnum<class "Motion.lvclass">, "Gantry"=w859:dbl[])  [unwired: 4 in, 2 out]
        n284 = Subtract(x=w859, y=w858) -> (x-y=w857:dbl[])
        n285 = call "Joystick and Camera SHIH VPC- external Connection.vi"("Motion in"=w869, "XYZTheta"=w857, "Measurement Point"="Measure the touch spot with camera") -> ("Motion out"=w865:refnum<class "Motion.lvclass">, "Gantry"=w868:dbl[])  [unwired: 4 in, 2 out]
        n286 = Subtract(x=w859, y=w868) -> (x-y=w867:dbl[])
        n287 = call-poly <vilib>:"Write Delimited Spreadsheet.vi"("file path (dialog if empty)"=path "D:/INTT/V1/Assembly Data/Tool Offsets/Dispense Tip Offset.txt", "1D data"=w867, "append to file? (new file:F)"=FALSE) -> ()  [unwired: 11 in, 2 out]
      }
      event "Pick and place": Value Change {
        (unwired) "PICK and PLACE samples ..." ("String")
        n288 = event-data() -> ()  [unwired: 1 in, 6 out]
        n289 = Build Array(0.0 ("element"), 0.0 ("element"), 0.0 ("element"), 0.0 ("element")) -> (w903:dbl[])
        n290 = Build Array(0.0 ("element"), 0.0 ("element"), 0.0 ("element"), 0.0 ("element")) -> (w902:dbl[])
        n291 = case shown="True" w897 {
          tunnel: w922 -> [w1074 w1096]
          tunnel: [w1073 w1095] -> _
          frame False {
            n292 = Array Subset(array=w1074, index (row)=0 ("index"), length (row)=1 ("length")) -> (w1076:dbl[][])  [unwired: 2 in]
            n293 = Build Array(11.75 ("element"), 173.55 ("element"), 0.0 ("element"), 0.0 ("element")) -> (w1080:dbl[])
            n294 = Reshape Array(w1076, 4 ("dimension size")) -> (w1075:dbl[])
            n295 = Add(x=w1080, y=w1075) -> (x+y=w1073:dbl[])
          }
          frame True {
            n296 = Array Subset(array=w1096, index (row)=0 ("index"), length (row)=1 ("length")) -> (w1086:dbl[][])  [unwired: 2 in]
            n297 = Build Array(11.75 ("element"), 56.85 ("element"), 0.0 ("element"), 0.0 ("element")) -> (w1090:dbl[])
            n298 = Reshape Array(w1086, 4 ("dimension size")) -> (w1085:dbl[])
            n299 = Add(x=w1090, y=w1085) -> (x+y=w1095:dbl[])
          }
        }
        n300 = Not(x=w897) -> (.not. x?=w896:bool)
        n301 = case shown="True" w896 {
          tunnel: w903 -> [w1067 w1070]
          tunnel: w902 -> [w1068 w1071]
          tunnel: [w1069 w1072] -> w901
          frame False {
            n302 = Build Array(w1068, w1067) -> (w1069:dbl[][])
          }
          frame True {
            n303 = Build Array(w1070, w1071) -> (w1072:dbl[][])
          }
        }
        n304 = for {
          tunnel: [w946] -> w895
          tunnel: w901 -> [w945] mode=indexing
          tunnel: w898 -> [w942] mode=indexing
          n305 = Index Array(array=w942, index=3) -> (element=w943:dbl)
          n306 = Multiply(x=w943, y=-1.0) -> (x*y=w941:dbl)
          n307 = Index Array(array=w945, index=0) -> (element=w952:dbl)
          n308 = Index Array(array=w945, index=1) -> (element=w951:dbl)
          n309 = call-poly <vilib>:"2D Cartesian Coordinate Rotation.vi"("theta"=w941, "y"=w951, "x"=w952) -> ("y out"=w954:dbl, "x out"=w953:dbl)  [unwired: 6 in, 1 out]
          n310 = Build Array(w953, w954, 0.0 ("element"), 0.0 ("element")) -> (w946:dbl[])
        }
        "?" <- w895
        n311 = Array Subset(array=w898, index (row)=0 ("index"), length (row)=1 ("length")) -> (w909:dbl[][])  [unwired: 2 in]
        n312 = Reshape Array(w909, 4 ("dimension size")) -> (w900:dbl[])
        n313 = Add(x=w895, y=w900) -> (x+y=w899:dbl[])
        "CT sum up" <- w899
        n314 = call-poly <vilib>:"Read Delimited Spreadsheet.vi"("file path (dialog if empty)"=path "D:/INTT/V1/Assembly Data/Tool Offsets/Bellows Tool Offset.txt", "number of rows (all:-1)"=-1) -> ("first row"=w937:dbl[])  [unwired: 8 in, 5 out]
        n315 = Index Array(array=w937, index #1=0 ("index"), index #2=1 ("index"), index #3=2 ("index")) -> (element #1=w933:dbl, element #2=w932:dbl, element #3=w931:dbl)
        n316 = for {
          N: 1 -> [_]
          tunnel: w940 -> [w965]
          tunnel: [w986] -> w930
          tunnel: w929 -> [w958] mode=indexing
          tunnel: [w974] -> w925
          tunnel: w926 -> [w964]
          tunnel: w933 -> [w988]
          tunnel: w932 -> [w987]
          tunnel: w931 -> [w985]
          tunnel: w918 -> [w980]
          tunnel: w924 -> [w967]
          tunnel: w899 -> [w966]
          tunnel: w920 -> [w962]
          tunnel: w898 -> [w957]
          tunnel: w895 -> [w956]
          w976 = 0 ("Write")
          w979 = TRUE ("Write Value")
          # "putback pickup tool"
          # "pickup tool"
          # "pickup tool height offset"
          # "Pick up PICKUP TOOL"
          # "Pick up CHIPs/Sensor and place on HDI"
          n317 = Build Array(w988, w987, w985, 0.0 ("element")) -> (w959:dbl[])
          n318 = Add(x=w958, y=w959) -> (x+y=w960:dbl[])
          n319 = call "XYZTheta-2Zspeed Go.vi"("XYZTheta In"=w960, "Motion in"=w965) -> ("error out"=w963:errorcluster, "Motion out"=w961:refnum<class "Motion.lvclass">)  [unwired: 7 in, 1 out]
          n320 = call "WriteReadWait.vi"("Read Value"=w979, "Write Value"=w979, "error in (no error)"=w963, "Read"=w976, "Write"=w976, "I-O in"=w964) -> ("error out"=w978:errorcluster, "I-O out"=w977:refnum<class "NI-DAQ.lvclass">)  [unwired: 4 in]
          n321 = Replace Array Subset(array=w959, new element=-10.5 ("t"), index=2) -> (w983:dbl[])
          n322 = for {
            N: w980 -> [_]
            tunnel: w961 -> [w1009]
            tunnel: w983 -> [w1008]
            tunnel: w978 -> [w1007]
            tunnel: [w1006] -> w989
            tunnel: w977 -> [w1005]
            tunnel: [w1004] -> w975
            tunnel: [w1003] -> w982
            tunnel: w967 -> [w1000]
            tunnel: w966 -> [w997]
            tunnel: w962 -> [w999] mode=indexing
            tunnel: w957 -> [w998] mode=indexing
            tunnel: w956 -> [w996]
            n323 = flat-sequence {
              tunnel: [w1031] -> w1010
              tunnel: w1009 -> [w1030]
              tunnel: w1008 -> [w1029]
              tunnel: w1007 -> [w1027]
              tunnel: w1005 -> [w1021]
              tunnel: [w1026] -> w1002
              tunnel: [w1013] -> w1001
              tunnel: w1000 -> [w1012]
              tunnel: w997 -> [w1024]
              tunnel: [w1015] -> _
              tunnel: w996 -> [w1015]
              tunnel: [w1015] -> w995
              tunnel: w1010 -> [w1055]
              tunnel: [w1066] -> w1006
              tunnel: [w1065] -> _
              tunnel: [w1061] -> w1004
              tunnel: [w1035] -> w1003
              tunnel: w1002 -> [w1063]
              tunnel: w1001 -> [w1059]
              tunnel: w999 -> [w1060]
              tunnel: w998 -> [_]
              tunnel: w997 -> [w1037]
              tunnel: w995 -> [_]
              frame #0 {
                w1019 = FALSE ("Write Value")
                w1025 = TRUE ("Write Value")
                w1011 = 1 ("Write")
                # "pickup module"
                # "release module"
                # "pickup sample from tray"
                n324 = Add(x=w1024, y=w1029) -> (x+y=w1028:dbl[])
                n325 = call "XYZTheta-2Zspeed Go.vi"("error in (no error)"=w1027, "XYZTheta In"=w1028, "Motion in"=w1030) -> ("error out"=w1022:errorcluster, "Motion out"=w1031:refnum<class "Motion.lvclass">)  [unwired: 6 in, 1 out]
                n326 = call "Time Delay"("error in (no error)"=w1022) -> ("error out"=w1016:errorcluster)  [unwired: 10 in]
                n327 = call "0"("error in (no error)"=w1016) -> ("error out"=w1017:errorcluster)  [unwired: 9 in, 1 out]
                n328 = call "WriteReadWait.vi"("Read Value"=w1019, "Write Value"=w1019, "error in (no error)"=w1017, "Read"=w1012, "Write"=w1012, "I-O in"=w1021) -> ("error out"=w1018:errorcluster, "I-O out"=w1020:refnum<class "NI-DAQ.lvclass">)  [unwired: 4 in]
                n329 = call "Time Delay3"("error in (no error)"=w1018) -> ("error out"=w1023:errorcluster)  [unwired: 10 in]
                n330 = call "WriteReadWait.vi"("Read Value"=w1025, "Write Value"=w1025, "error in (no error)"=w1023, "Read"=w1011, "Write"=w1011, "I-O in"=w1020) -> ("error out"=w1014:errorcluster, "I-O out"=w1026:refnum<class "NI-DAQ.lvclass">)  [unwired: 4 in]
                n331 = call "Delay5"("error in (no error)"=w1014) -> ("error out"=w1013:errorcluster)  [unwired: 10 in]
              }
              frame #1 {
                w1062 = 1 ("Write")
                w1064 = FALSE ("Write Value")
                # "lift for chip/sensor thickness"
                # "place sample on HDI"
                n332 = Add(x=w1060, y=dbl[] [0.0, 0.0, -16.0, 0.0]) -> (x+y=w1053:dbl[])
                n333 = call-dynamic "Get Current Position.vi"("Motion in"=w1055) -> ("XYZTheta Out"=w1051:dbl[], "Motion out"=w1054:refnum<class "Motion.lvclass">)  [unwired: 8 in, 1 out]
                "gantry position test" <- w1051
                n334 = Array Subset(array=w1037, index=0, length=2) -> (w1040:dbl[])
                n335 = Build Array (concatenate)(w1040, 0.0 ("element"), 0.0 ("element")) -> (w1039:dbl[])
                n336 = Subtract(x=w1053, y=w1039) -> (x-y=w1052:dbl[])
                "displacement" <- w1052
                n337 = Array Subset(array=w1051, index=0, length=2) -> (w1046:dbl[])
                n338 = Build Array (concatenate)(w1046, 0.0 ("element"), 0.0 ("element")) -> (w1045:dbl[])
                n339 = Add(x=w1045, y=w1052) -> (x+y=w1033:dbl[])
                n340 = Add(x="offset", y=w1033) -> (x+y=w1032:dbl[])
                "gantry target position" <- w1032
                n341 = call "XYZTheta-2Zspeed Go.vi"("error in (no error)"=w1059, "XYZTheta In"=w1032, "Motion in"=w1054) -> ("error out"=w1058:errorcluster, "XYZTheta Out"=w1065:dbl[], "Motion out"=w1066:refnum<class "Motion.lvclass">)  [unwired: 6 in]
                n342 = call "1"("error in (no error)"=w1058) -> ("error out"=w1057:errorcluster)  [unwired: 9 in, 1 out]
                n343 = call "Time Delay6"("error in (no error)"=w1057) -> ("error out"=w1056:errorcluster)  [unwired: 10 in]
                n344 = call "WriteReadWait.vi"("Read Value"=w1064, "Write Value"=w1064, "error in (no error)"=w1056, "Read"=w1062, "Write"=w1062, "I-O in"=w1063) -> ("error out"=w1036:errorcluster, "I-O out"=w1061:refnum<class "NI-DAQ.lvclass">)  [unwired: 4 in]
                n345 = call "Time Delay4"("error in (no error)"=w1036) -> ("error out"=w1035:errorcluster)  [unwired: 10 in]
              }
            }
          }
          n346 = call "XYZTheta-2Zspeed Go.vi"("error in (no error)"=w982, "XYZTheta In"=w960, "Motion in"=w989) -> ("error out"=w970:errorcluster, "Motion out"=w993:refnum<class "Motion.lvclass">)  [unwired: 6 in, 1 out]
          n347 = call "Time Delay9"("error in (no error)"=w970) -> ("error out"=w972:errorcluster)  [unwired: 10 in]
          n348 = call-dynamic "Digital Write 1 Channel.vi"("DAQ Module"=0, "error constant"=w972, "Value"=FALSE, "Channel"=0, "NI-DAQ.lvclass"=w975) -> ("error IO"=w971:errorcluster, "NI-DAQ.lvclass 2"=w974:refnum<class "NI-DAQ.lvclass">)  [unwired: 5 in]
          n349 = call "Time Delay10"("error in (no error)"=w971) -> ("error out"=w990:errorcluster)  [unwired: 10 in]
          n350 = call-dynamic "Z Go.vi"("error in (no error)"=w990, "Speed"=10.0, "Position"=0.0 ("new element/subarray"), "Motion in"=w993) -> ("Motion out"=w986:refnum<class "Motion.lvclass">)  [unwired: 6 in, 1 out]
        }
      }
      event "GOTO": Value Change {
        (unwired) "GOING to a position" ("String")
        n351 = event-data() -> ()  [unwired: 1 in, 6 out]
        n352 = call "XYZTheta Go.vi"("XYZTheta In"="Parking position", "Motion in"=w1105) -> ("Motion out"=w1103:refnum<class "Motion.lvclass">)  [unwired: 7 in, 2 out]
      }
      event "READ Position": Value Change {
        n353 = event-data() -> ()  [unwired: 1 in, 6 out]
        n354 = call-dynamic "Get Current Position.vi"("Motion in"=w1126) -> ("XYZTheta Out"=→"Gantry current position":dbl[], "Motion out"=w1125:refnum<class "Motion.lvclass">)  [unwired: 8 in, 1 out]
      }
      event "HDI vacuum": Value Change {
        n355 = event-data() -> ()  [unwired: 1 in, 6 out]
        n356 = call "WriteReadWait.vi"("Read Value"="vacuum", "Write Value"="vacuum", "Read"=w1140, "Write"=w1140, "I-O in"=w1143) -> ("error out"=w1141:errorcluster, "I-O out"=w1130:refnum<class "NI-DAQ.lvclass">)  [unwired: 5 in]
        n357 = call "Time Delay2"("error in (no error)"=w1141) -> ()  [unwired: 10 in, 1 out]
      }
      event Timeout {
        n358 = event-data() -> ()  [unwired: 1 in, 3 out]
        n359 = call-dynamic "Digital Read 1 Channel.vi"("Read"=w1157, "NI-DAQ in"=w1158) -> ("Value"=→"Status":bool, "NI-DAQ out"=w1156:refnum<class "NI-DAQ.lvclass">)  [unwired: 7 in, 1 out]
      }
    }
    "Measured HDI size" <- w30
    "MPT positions on stave" <- w31
    "Stave mark" <- w29
    "measured HDI top-left position" <- w26
    n360 = feedback-in #1(w30) -> ()
    n361 = feedback-in #2(w29) -> ()
    n362 = feedback-in #3(w26) -> ()
    n363 = feedback-in #4(w15) -> ()
    n364 = feedback-in #5(w41) -> ()
    n365 = feedback-in #6(w38) -> ()
    n366 = feedback-in #7(w46) -> ()
    n367 = feedback-in #8(w12) -> ()
    n368 = feedback-in #9(w31) -> ()
    n369 = feedback-in #10(w47) -> ()
    n370 = feedback-in #11(w10) -> ()
    "# of tasks excuted" <- w43
  }
  n371 = call-dynamic "Disconnect.vi"("Controller in"=w4) -> ()  [unwired: 9 in, 1 out]
  n372 = call-dynamic "Disconnect.vi"("I-O in"=w1) -> ()  [unwired: 9 in, 1 out]
